vi "WF phase diversity_MATLAB_Correction_loop_AndorSDK_OneCorrApplyToAll_imq.vi"() -> ()   [LabVIEW 2018]
uses:
  <userlib>/WaveKit.lib/Controls/Wavefront Corrector states - ONE.ctl
  <userlib>/WaveKit.lib/Classes/WavefrontCorrector/WavefrontCorrector.lvclass
  <userlib>/WaveKit.lib/Classes/WavefrontCorrectorSet/WavefrontCorrectorSet.lvclass
  <vilib>/Analysis/1siggen.llb/Ramp Pattern by Samples.vi
  <vilib>/Utility/file.llb/Read From Spreadsheet File (DBL).vi
  <vilib>/Analysis/1siggen.llb/Ramp Pattern by Delta.vi
  <vilib>/Analysis/NI_AALBase.lvlib
panel:
  in  "Tab Control":T1(tab)
  in  "Offset command file":path=path "D:/SystemAlignment/system_aberration_20200206.dat"
  in  "Initial haso file":path=path "D:/SystemAlignment/system_aberration_residual_20191015.has"
  out "# of Phase":i32
  in  "Error in":errorcluster
  in  "DM configuration file":path=path "C:/Program Files (x86)/Imagine Optic/Configuration Files/WaveFrontCorrector_mirao52-e_0326.dat"
  out "DM Initial State":T2[](array[typedef])
  out "DM ActuatorsNumber":i32
  out "Error out":errorcluster
  in  "EMCCD trigger port":tag="Dev1/port0/line0"
  in  "Cooler set to Temperature":i32=-60
  in  "Trigger":u32(ring)=1 items=["Internal", "External"]
  out "Return from CheckTimings":u32
  out "Calculated Exposure Value":sgl format="%.2f"
  out "Return from SetTemperature":u32
  out "Cooling":i32
  out "Return from Initialize":u32
  out "Detector X Pixels":i32
  out "Detector Y Pixels":i32
  in  "Initialize EMCCD?":bool=TRUE
  in  "Turn off EMCCD when finished?":bool=TRUE
  in  "Initial Zer coeff":dbl[](array[numeric])=[0.2, 0.2]
  in  "Initial Zer index":dbl[](array[numeric])=[4.0, 5.0]
  out "Initial Zer coeff\nRandomly generated":dbl[](array[numeric])
  out "Initial Zer index (starting from 4)\nrandomly generated":dbl[](array[numeric])
  in  "aberration tolerance":dbl=0.1 format="%#_13g"
  in  "aberration threshold":dbl=0.25 format="%#_13g"
  in  "?":enum16{"input manually ", "randomly generated"}(ring)
  in  "max random order":i64=9
  in  "NOT YET: Data Acquisition Iteration #":i32=1
  in  "Zern index in 2":i32[](array[numeric])=[3, 4, 5, 6, 7, 8]
  in  "Zern coef in 2":sgl[](array[numeric])=[0.0, 0.0, 0.2, 0.0, 0.0, 0.0]
  in  "Zern index in 3":i32[](array[numeric])=[3, 4, 5, 6, 7, 8]
  in  "Zern coef in 3":sgl[](array[numeric])=[0.2, 0.0, 0.0, 0.0, 0.0, 0.0]
  in  "Zern index in 4":i32[](array[numeric])=[3, 4, 5, 6, 7, 8]
  in  "Zern coef in 4":sgl[](array[numeric])=[0.2, 0.0, 0.0, 0.0, 0.0, 0.0]
  in  "Zern index in 5":i32[](array[numeric])=[3, 4, 5, 6, 7, 8]
  in  "Zern coef in 5":sgl[](array[numeric])=[0.0, 0.0, 0.0, 0.0, 0.0, -0.2]
  in  "Andor Picture/notes save to path":path=path "D:/YD/test/test1"
  in  "base name":string="beads_test"
  in  "Pics/phase":dbl=2.0
  in  "camera exposure time (s)":string="0.02"
  in  "# of Phase":i32=5
  in  "COMMAND matrix path":path=path "D:/SystemAlignment/IM_20200224.aomi"
  in  "488 shutter":refnum<k7>(container)
  in  "?":bool
  out "phase diversity file name":string
  out "Corrected Picture name":string
  in  "Z for correction (um) (10 steps=1um)":dbl format="%#_13g"
  in  "ASI stage VISA resource name":refnum<visa-resource-name>="COM5"
  in  "Z scanning range (um)":dbl format="%#_13g"
  in  "Z scanning step (um)":dbl format="%#_13g"
  out "Current Z in step":string="where z"
  in  "Background Value":u32=290
  in  "Run MATLAB or correction?":bool=TRUE
  in  "Keep Reconstructed Defocus component? 2":bool caption="Keep Reconstructed Defocus component?"
  in  "Number for average 2":u32=2
  in  "Zernike Order 2":u32=15
  in  "Iteration Number 2":u32=10
  in  "Gamma Value 2":dbl=1e-06
  in  "Crop Size of image 2":u32=512
  in  "Show Input 2":bool
  in  "Show Recon 2":bool=TRUE
  in  "Use GPU 2":bool=TRUE
  in  "Metrics Type":T3(ring)
  # "If Pics/phase is 2:\npicture order:\n\noffset+aberr *2\nphase diversity *8\n\nground truth *1\noffset+aberr *1\ncorrected *2 but the last one cannot be seen in imagej"
  # "Randomly Generate Initial Zernike, enter here:"
  # "Manually input, enter here:"
  # "Andor Camera Settings"
  # "z-stack is from (Z_for_correction-Z_scanning_range) to (Z_for_correction+Z_scanning_range)"
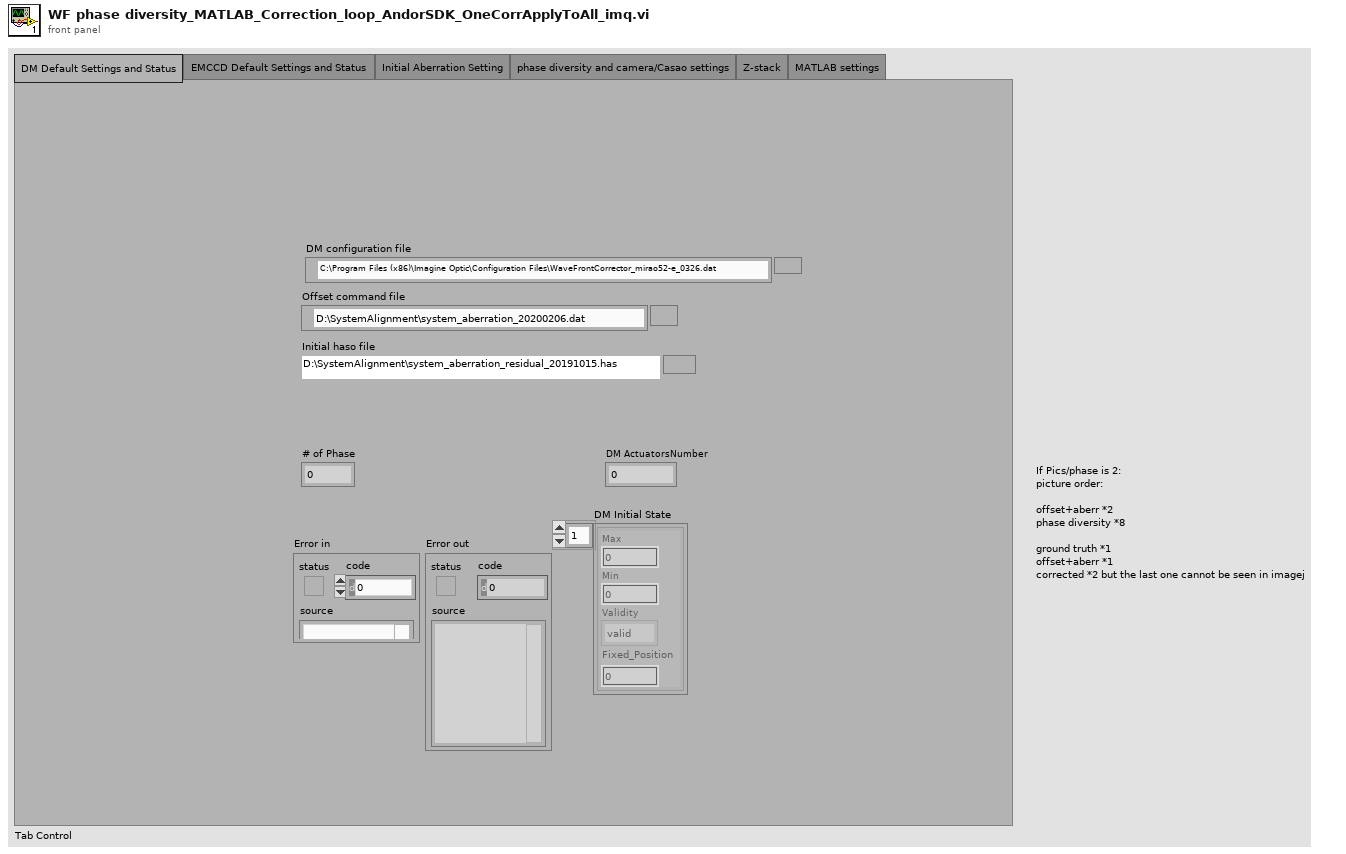
[diagram p1: front panel]
types:
  T1 = enum32{"DM Default Settings and Status", "EMCCD Default Settings and Status ", "Initial Aberration Setting", "phase diversity and camera/Casao settings", "Z-stack", "MATLAB settings"}
  T2 = typedef "Wavefront Corrector states - ONE.ctl" = cluster{"Max":sgl, "Min":sgl, "Validity":enum16{"valid", "fixed", "invalid"}, "Fixed_Position":sgl}
  T3 = enum16{" ", "max intensity", "mean intensity", "RMS contrast", "sharpness - image domain", "sharpness - spectral domain 1: 0~r0", "sharpness - spectral domain 2: 0.1*r0~0.5*r0", "norm DCT  - spectral domain 3: 0~r0"}
  T4 = typedef "Error Code Enum typedef.ctl" = enum32{"N/A (0)", "DRV_ERROR_CODES", "DRV_SUCCESS", "DRV_VXDNOTINSTALLED", "DRV_ERROR_SCAN", "DRV_ERROR_CHECK_SUM", "DRV_ERROR_FILELOAD", "DRV_UNKNOWN_FUNC", "DRV_ERROR_VXD_INIT", "DRV_ERROR_ADDRESS", "DRV_ERROR_PAGELOCK", "DRV_ERROR_PAGEUNLOCK", "DRV_ERROR_BOARDTEST", "DRV_ERROR_ACK", "DRV_ERROR_UP_FIFO", "DRV_ERROR_PATTERN", "N/A (16)", "DRV_ACQUISITION_ERRORS", "DRV_ACQ_BUFFER", "DRV_ACQ_DOWNFIFO_FULL", "DRV_PROC_UNKONWN_INSTRUCTION", "DRV_ILLEGAL_OP_CODE", "DRV_KINETIC_TIME_NOT_MET", "DRV_ACCUM_TIME_NOT_MET", "DRV_NO_NEW_DATA", "N/A (25)", "DRV_SPOOLERROR", "N/A (27)", "N/A (28)", "N/A (29)", "N/A (30)", "N/A (31)", "N/A (32)", "DRV_TEMPERATURE_CODES", "DRV_TEMPERATURE_OFF", "DRV_TEMPERATURE_NOT_STABILIZED", "DRV_TEMPERATURE_STABILIZED", "DRV_TEMPERATURE_NOT_REACHED", "DRV_TEMPERATURE_OUT_RANGE", "DRV_TEMPERATURE_NOT_SUPPORTED", "DRV_TEMPERATURE_DRIFT", "N/A (41)", "N/A (42)", "N/A (43)", "N/A (44)", "N/A (45)", "N/A (46)", "N/A (47)", "N/A (48)", "DRV_GENERAL_ERRORS", "DRV_INVALID_AUX", "DRV_COF_NOTLOADED", "DRV_FPGAPROG", "DRV_FLEXERROR", "DRV_GPIBERROR", "N/A (55)", "N/A (56)", "N/A (57)", "N/A (58)", "N/A (59)", "N/A (60)", "N/A (61)", "N/A (62)", "N/A (63)", "DRV_DATATYPE", "DRV_DRIVER_ERRORS", "DRV_P1INVALID", "DRV_P2INVALID", "DRV_P3INVALID", "DRV_P4INVALID", "DRV_INIERROR", "DRV_COFERROR", "DRV_ACQUIRING", "DRV_IDLE", "DRV_TEMPCYCLE", "DRV_NOT_INITIALIZED", "DRV_P5INVALID", "DRV_P6INVALID", "DRV_INVALID_MODE", "DRV_INVALID_FILTER", "DRV_I2CERRORS", "DRV_I2CDEVNOTFOUND", "DRV_I2CTIMEOUT", "DRV_P7INVALID", "N/A (84)", "N/A (85)", "N/A (86)", "N/A (87)", "N/A (88)", "N/A (89)", "DRV_IOCERROR", "DRV_VRMVERSIONERROR"}
  T5 = typedef "NI_Matrix.lvlib/RealMatrix.ctl" = dbl[][]
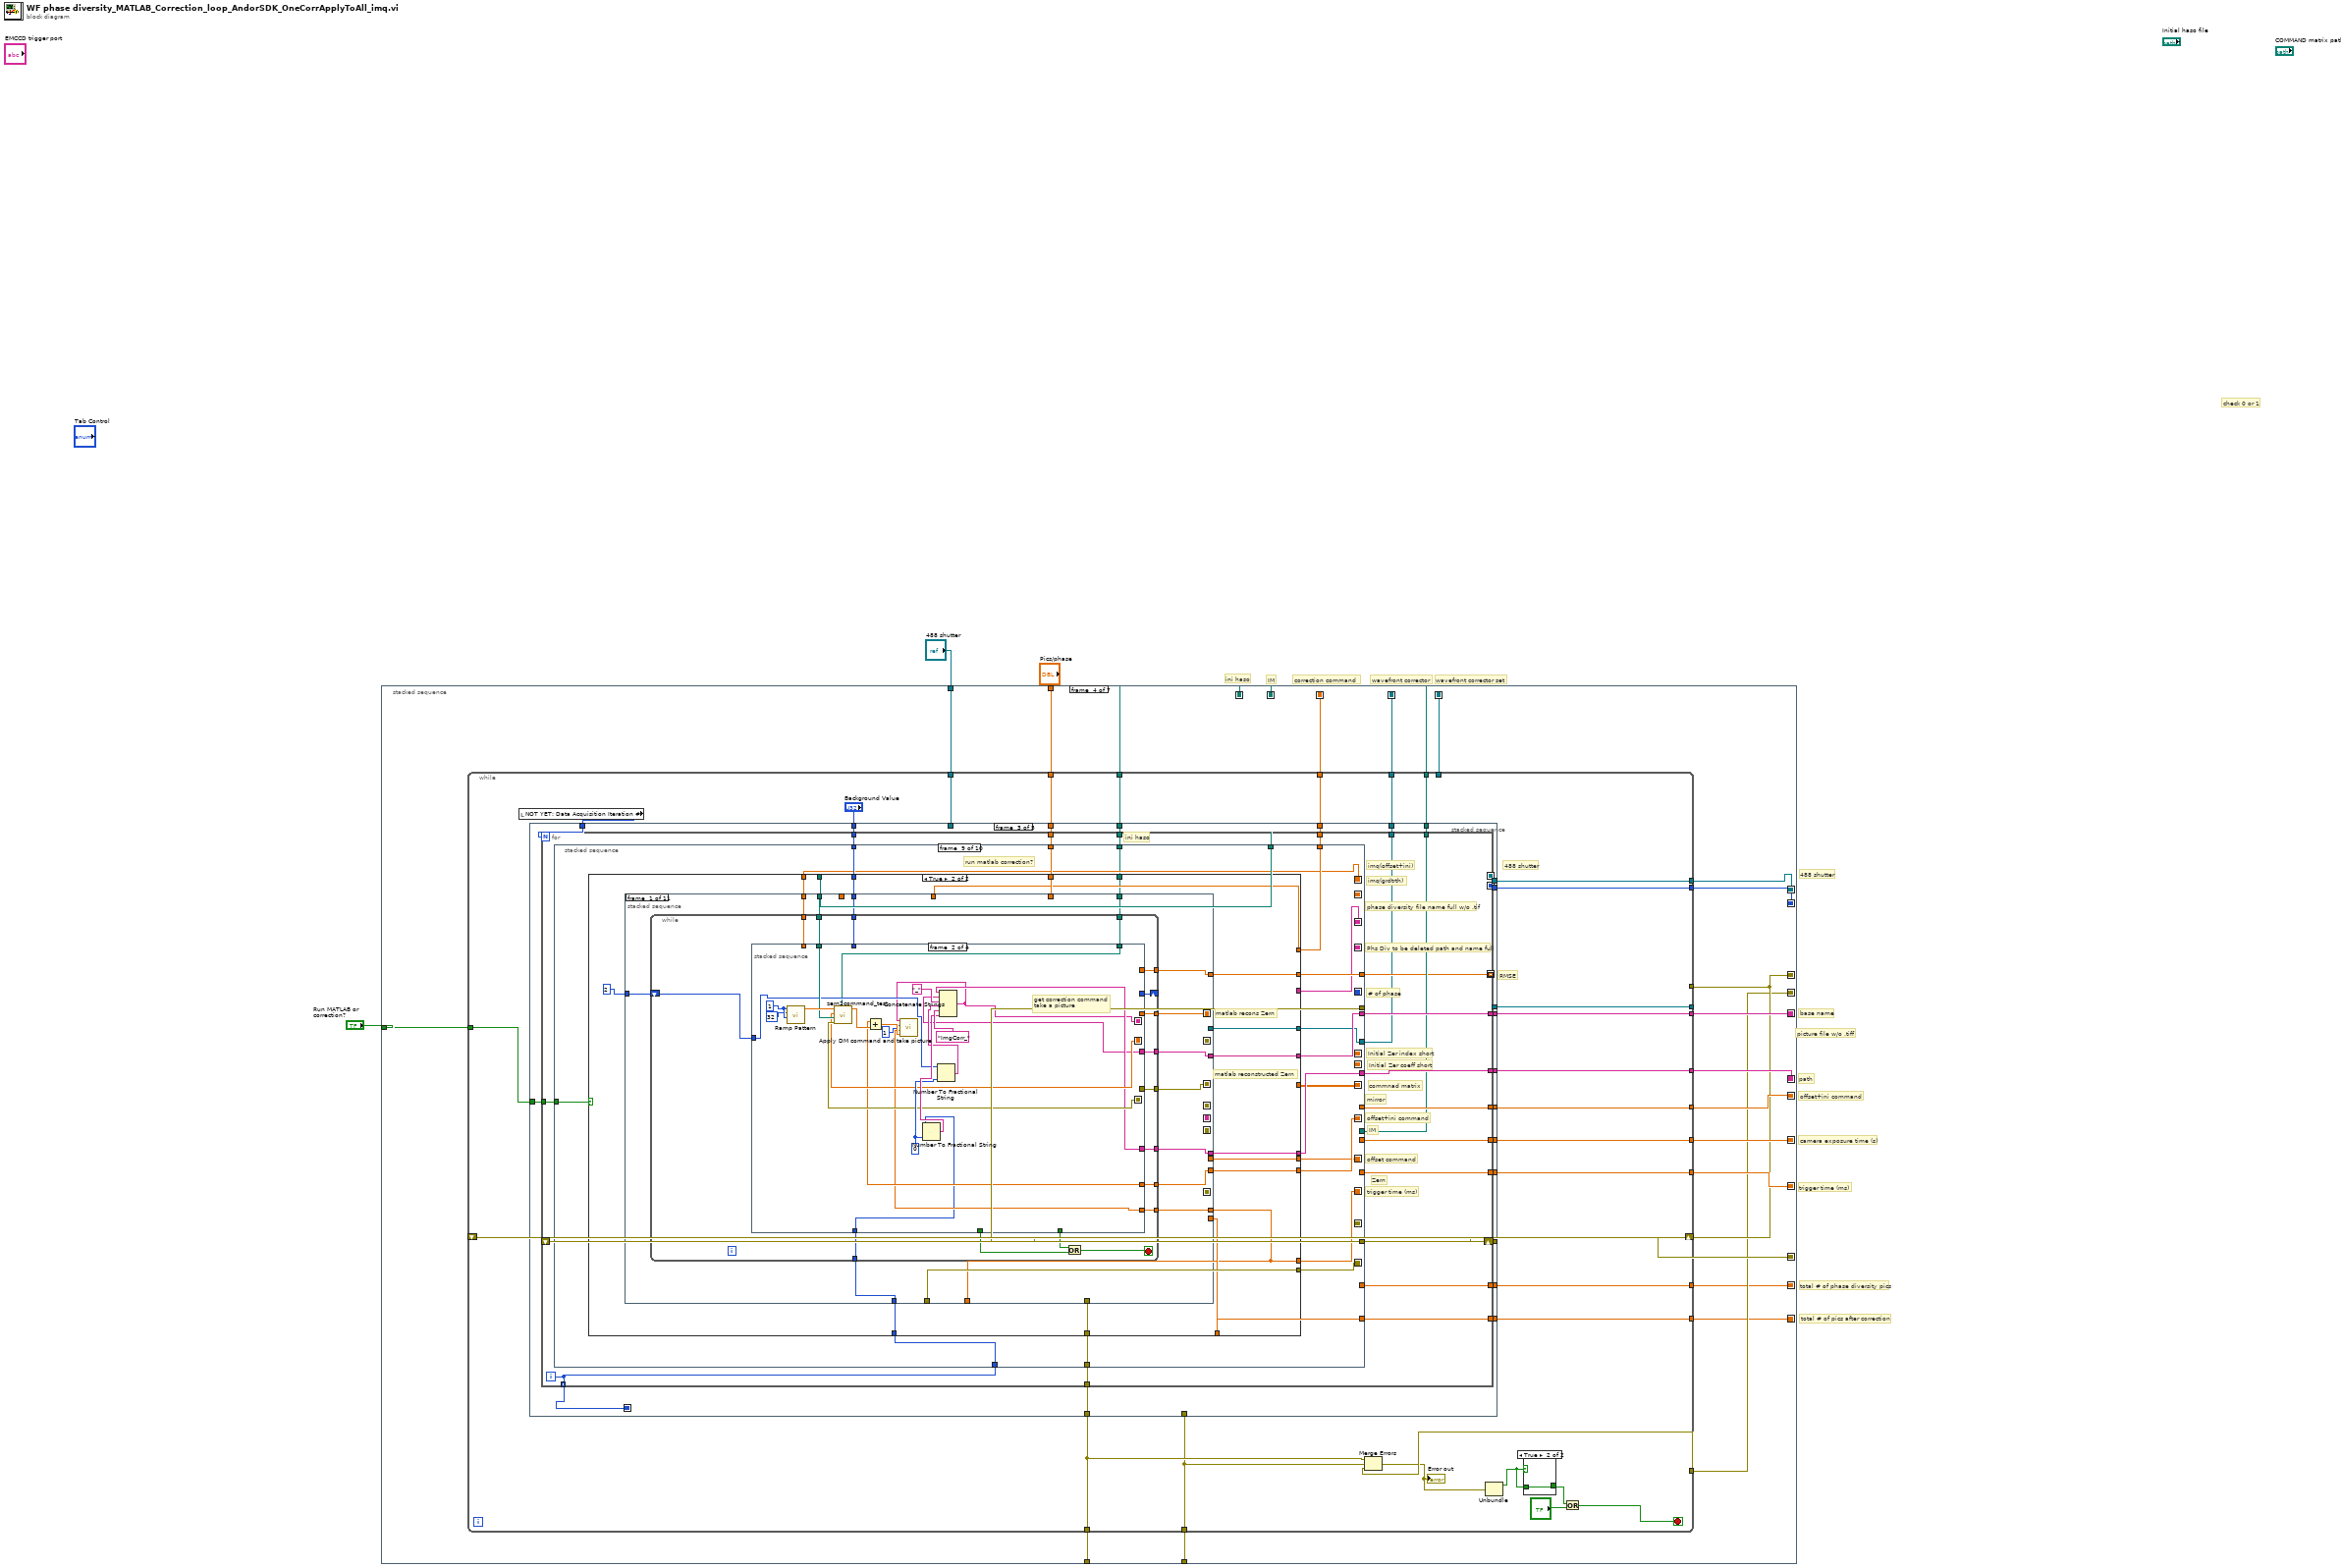
[diagram p0: block diagram]
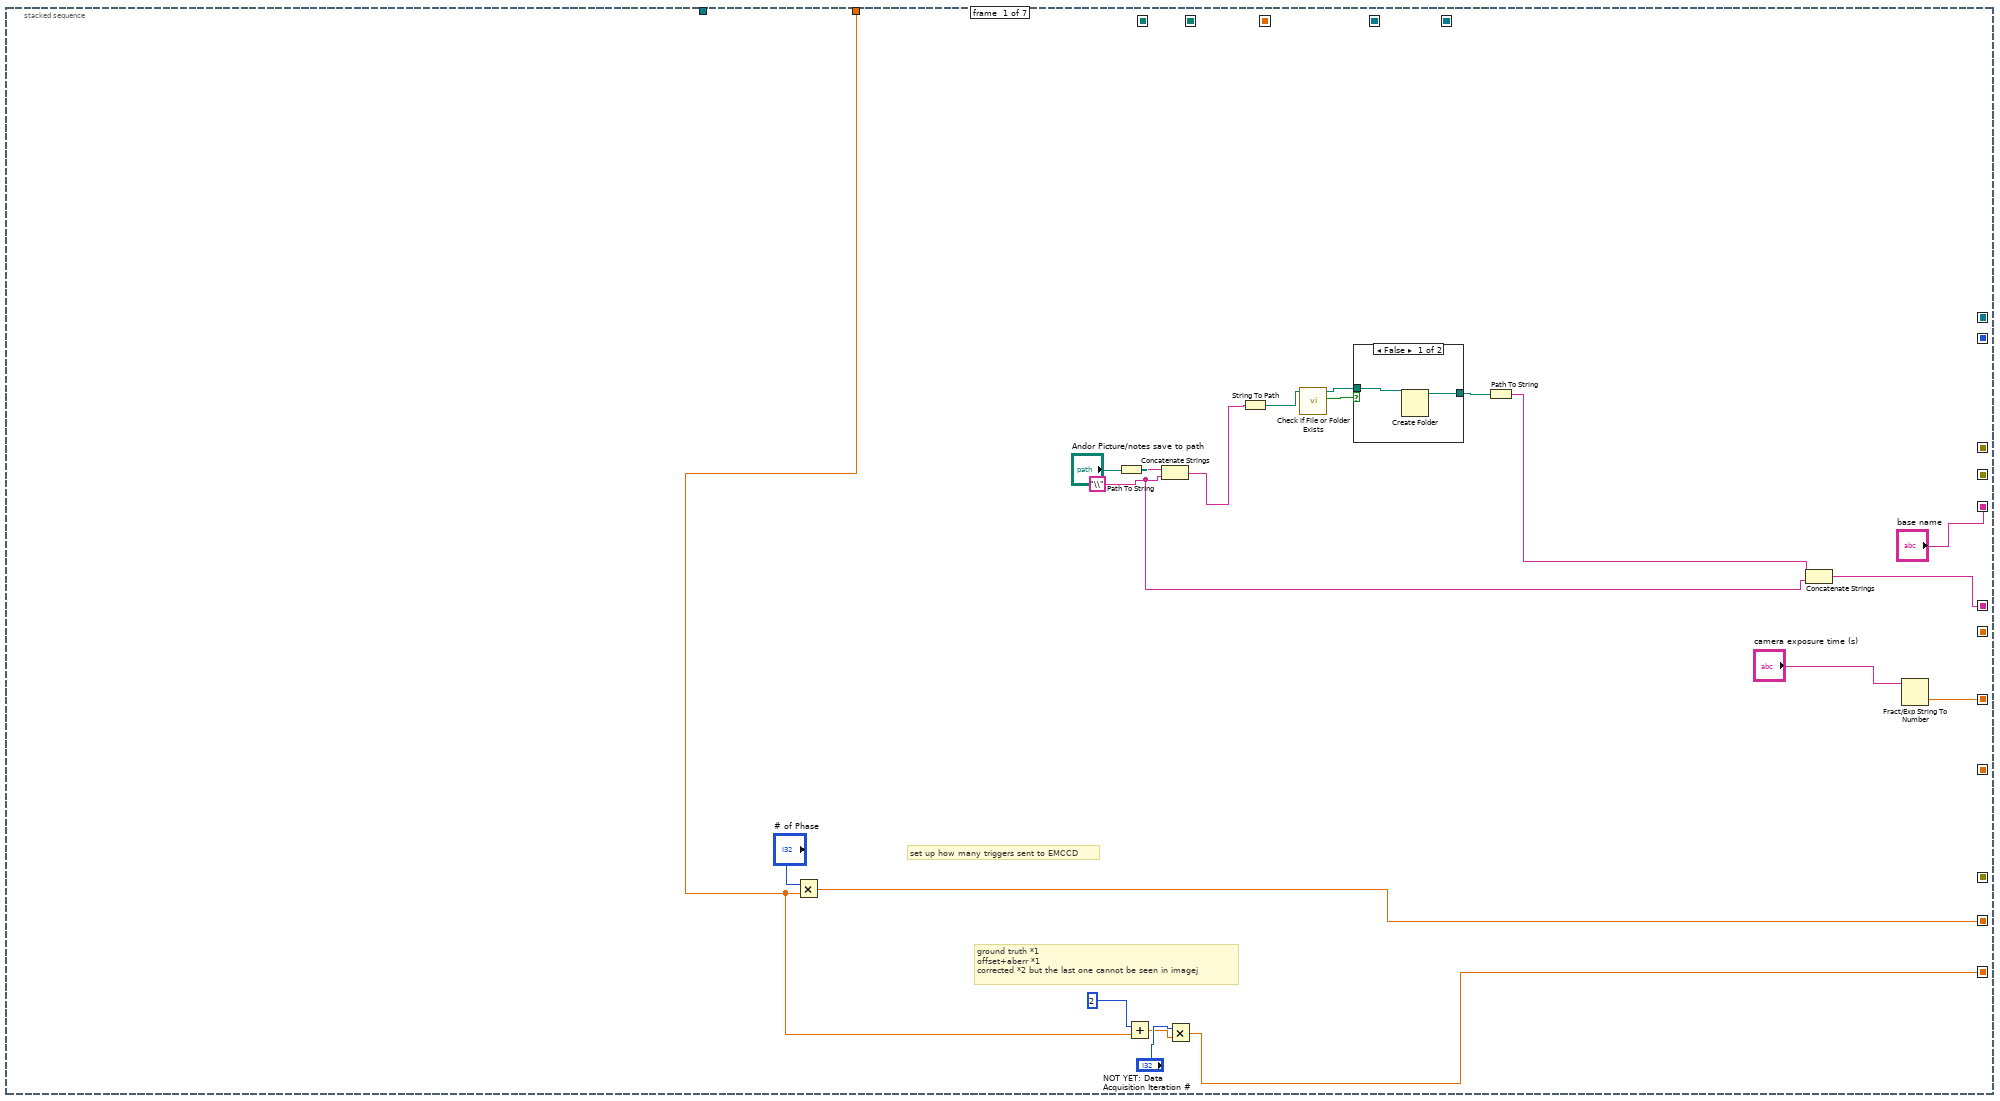
[diagram p2: hidden frame]
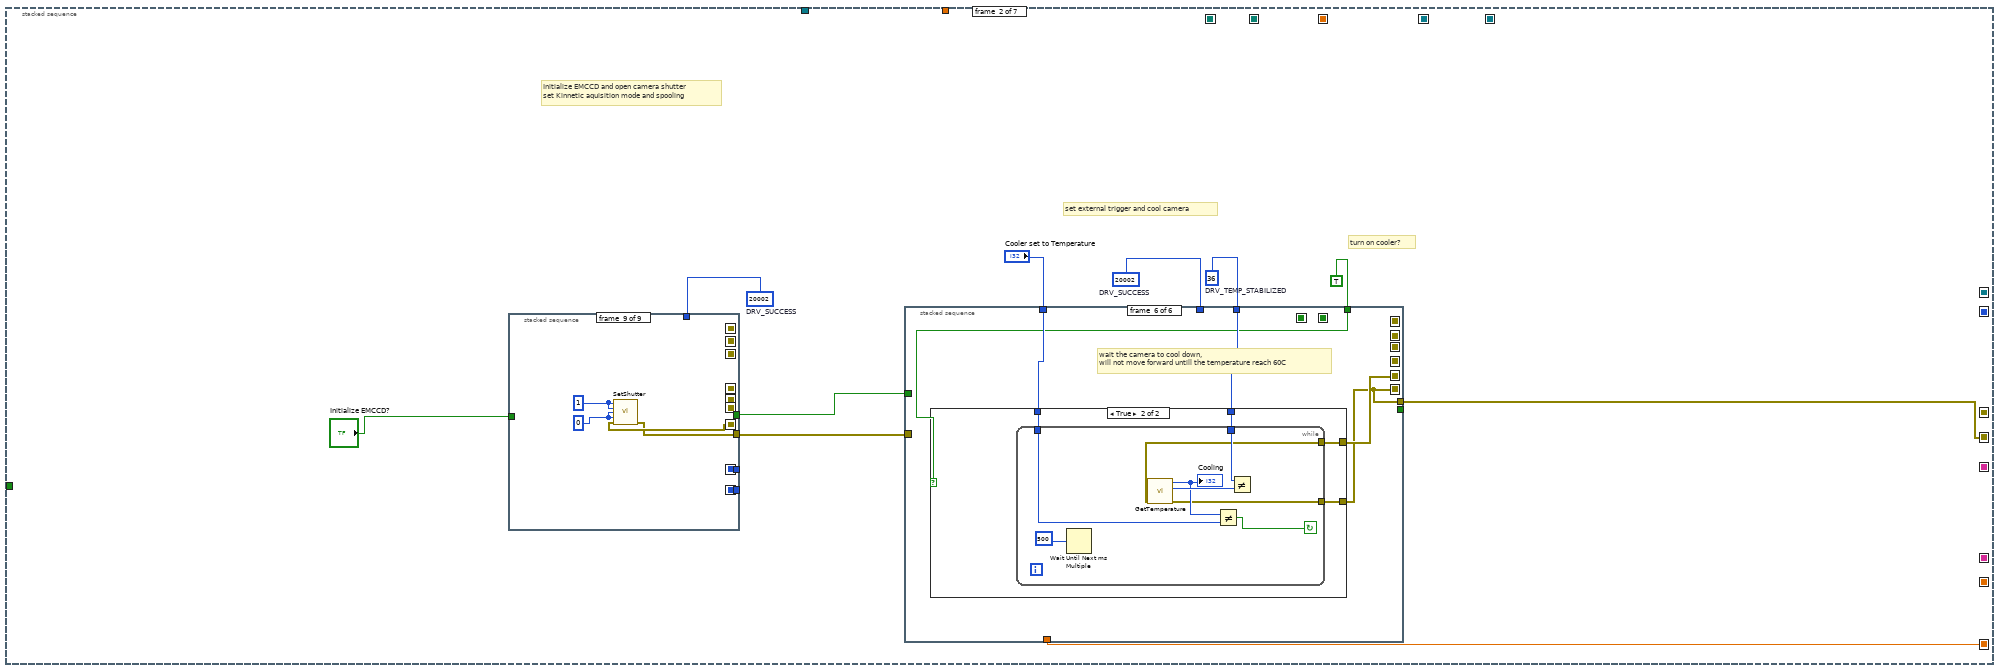
[diagram p4: hidden frame]
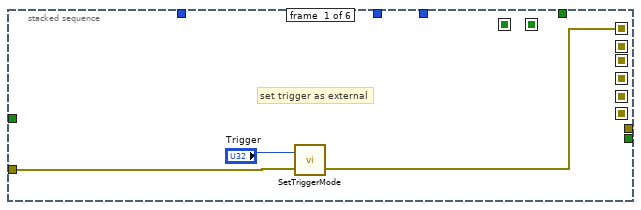
[diagram p5: hidden frame]
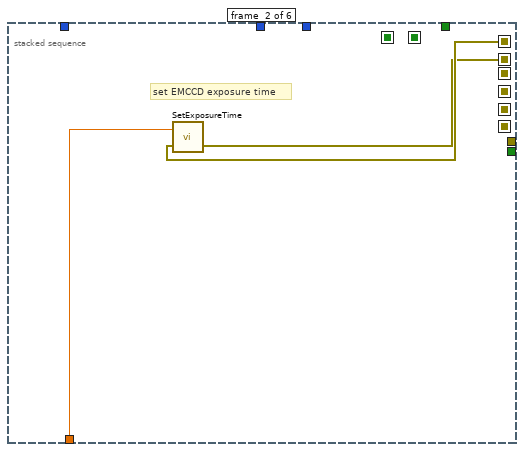
[diagram p6: hidden frame]
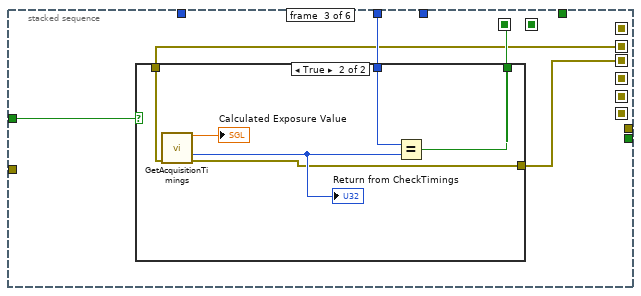
[diagram p7: hidden frame]
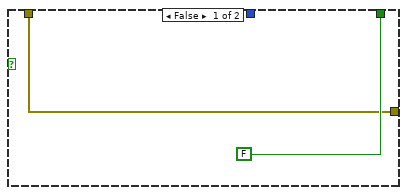
[diagram p8: hidden frame]
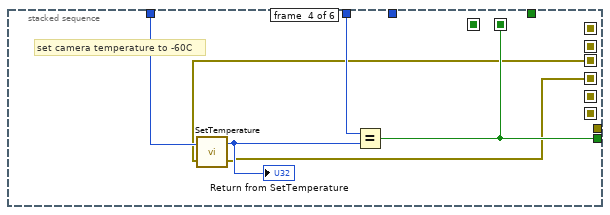
[diagram p9: hidden frame]
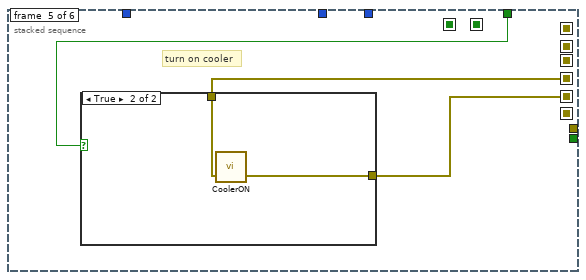
[diagram p10: hidden frame]
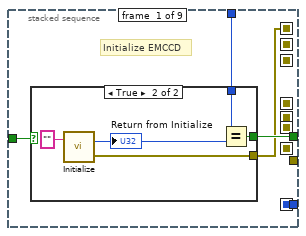
[diagram p13: hidden frame]
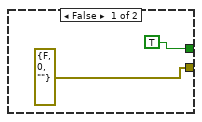
[diagram p14: hidden frame]
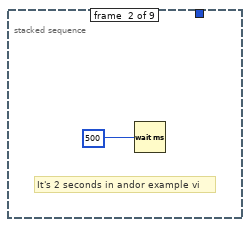
[diagram p15: hidden frame]
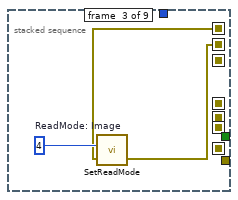
[diagram p16: hidden frame]
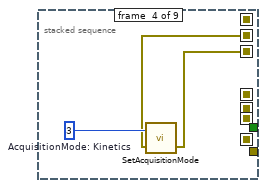
[diagram p17: hidden frame]
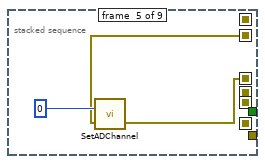
[diagram p18: hidden frame]
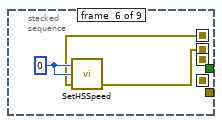
[diagram p19: hidden frame]
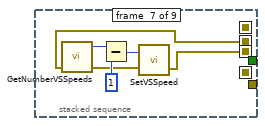
[diagram p20: hidden frame]
diagram:
  # "correction command"
  # "total # of phase diversity pics"
  # "picture file w/o .tiff"
  # "total # of pics after correction"
  # "wavefront corrector set"
  # "wavefront corrector"
  # "488 shutter"
  # "trigger time (ms)"
  # "offset+ini command"
  # "camera exposure time (s)"
  # "IM"
  # "ini haso"
  # "path"
  # "base name"
  # "check 0 or 1"
  n1 = stacked-sequence {
    seq-local: [w4 _ _ _ _ _ _] -> [_ _ _ w165 w746 _ _]
    seq-local: ["base name" _ _ _ _ _ _] -> [_ _ _ w164 w745 _ _]
    seq-local: [_ _ w144 _ _ _ _] -> [_ _ _ w163 _ _ _]
    seq-local: [_ _ w143 _ _ _ _] -> [_ _ _ w158 _ _ _]
    seq-local: [w18 _ _ _ _ _ _] -> [_ w29 _ w162 _ _ _]
    seq-local: [_ _ w128 _ _ _ _] -> [_ _ _ w150 _ _ _]
    seq-local: [_ _ _ w161 _ _ _] -> [_ _ _ _ _ _ _]
    seq-local: [_ _ _ w160 _ _ _] -> [_ _ _ _ w742 _ _]
    seq-local: [_ _ _ w159 _ _ _] -> [_ _ _ _ _ _ w828]
    seq-local: [_ _ _ w153 _ _ _] -> [_ _ _ _ w754 _ _]
    seq-local: [_ _ _ w156 _ _ _] -> [_ _ _ _ w753 _ _]
    seq-local: [_ _ w127 _ _ _ _] -> [_ _ _ w151 w751 _ w830]
    seq-local: [_ _ w126 _ _ _ _] -> [_ _ _ w149 _ _ w829]
    seq-local: [w15 _ _ _ _ _ _] -> [_ _ _ w146 _ _ _]
    seq-local: [_ w30 _ _ _ _ _] -> [_ _ _ w148 _ _ _]
    seq-local: [w14 _ _ _ _ _ _] -> [_ _ _ w147 _ _ _]
    seq-local: [_ _ _ w145 _ _ _] -> [_ _ _ _ w752 _ _]
    tunnel: "Pics/phase" -> [w12 _ _ w166 _ _ _]
    tunnel: "Run MATLAB or correction?" -> [_ _ _ w157 _ _ _]
    tunnel: [_ _ _ w155 _ _ _] -> _
    tunnel: [_ _ _ w154 _ _ _] -> _
    tunnel: "488 shutter" -> [_ _ _ w152 _ _ w831]
    frame #0 {
      w5 = "\\"
      # "set up how many triggers sent to EMCCD"
      # "ground truth *1\noffset+aberr *1\ncorrected *2 but the last one cannot be seen in imagej"
      n2 = Multiply(x="# of Phase", y=w12) -> (x*y=w14:dbl)
      n3 = Path To String(path="Andor Picture/notes save to path") -> (string=w20:string)
      n4 = Add(x=2, y=w12) -> (x+y=w16:dbl)
      n5 = Concatenate Strings(w20, w5) -> (w7:string)
      n6 = Multiply(x="NOT YET: Data Acquisition Iteration #", y=w16) -> (x*y=w15:dbl)
      n7 = String To Path(string=w7) -> (path=w11:path)
      n8 = call <vilib>:"Check if File or Folder Exists.vi"("path"=w11) -> ("file or folder exists?"=w9:bool, "dup path"=w10:path)  [unwired: 8 in, 1 out]
      n9 = case shown="False" w9 {
        tunnel: w10 -> [w25 w26]
        tunnel: [w24 w26] -> w8
        frame False {
          n10 = Create Folder(path (use dialog)=w25) -> (created path=w24:path)  [unwired: 2 in, 2 out]
        }
        frame True {
        }
      }
      n11 = Path To String(path=w8) -> (string=w6:string)
      n12 = Concatenate Strings(w6, w5) -> (w4:string)
      n13 = Fract/Exp String To Number(string="camera exposure time (s)") -> (number=w18:dbl)  [unwired: 3 in, 1 out]
    }
    frame #1 {
      w32 = 36  # DRV_TEMP_STABILIZED
      w34 = 20002  # DRV_SUCCESS
      w36 = 20002  # DRV_SUCCESS
      # "turn on cooler?"
      # "set external trigger and cool camera"
      # "Initialize EMCCD and open camera shutter\nset Kinnetic aquisition mode and spooling"
      n14 = stacked-sequence {
        seq-local: [_ _ _ _ _ _ _ w120 _] -> [_ _ _ _ _ _ _ _ _]
        seq-local: [_ _ _ _ _ _ _ w119 _] -> [_ _ _ _ _ _ _ _ _]
        seq-local: [w87 _ _ _ _ _ _ _ _] -> [_ _ w99 _ _ _ _ _ _]
        seq-local: [_ _ w98 _ _ _ _ _ _] -> [_ _ _ w102 _ _ _ _ _]
        seq-local: [_ _ _ w101 _ _ _ _ _] -> [_ _ _ _ w104 _ _ _ _]
        seq-local: [_ _ _ _ w105 _ _ _ _] -> [_ _ _ _ _ w108 _ _ _]
        seq-local: [_ _ _ _ _ w107 _ _ _] -> [_ _ _ _ _ _ w112 _ _]
        seq-local: [_ _ _ _ _ _ w110 _ _] -> [_ _ _ _ _ _ _ w118 _]
        seq-local: [_ _ _ _ _ _ _ w116 _] -> [_ _ _ _ _ _ _ _ w123]
        tunnel: w36 -> [w89 _ _ _ _ _ _ _ _]
        tunnel: [w88 _ _ _ _ _ _ _ _] -> w35
        tunnel: [_ _ _ _ _ _ _ w120 _] -> _
        tunnel: [_ _ _ _ _ _ _ w119 _] -> _
        tunnel: [_ _ _ _ _ _ _ _ w122] -> w31
        tunnel: "Initialize EMCCD?" -> [w86 _ _ _ _ _ _ _ _]
        frame #0 {
          # "Initialize EMCCD"
          n15 = case shown="True" w86 {
            tunnel: w89 -> [_ w94]
            tunnel: [TRUE w93] -> w88
            tunnel: [errorcluster {"status"=FALSE, "code"=0, "source"=""} ("Error in 2") w92] -> w87
            frame False {
            }
            frame True {
              n16 = call <userlib>:"Initialize.vi"("directory (\"\")"="" ("directory (\"\")")) -> ("error out"=w92:errorcluster, "DLL error code"=w96:u32)  [unwired: 1 in]
              "Return from Initialize" <- w96
              n17 = Equal?(x=w94, y=w96) -> (x = y?=w93:bool)
            }
          }
        }
        frame #1 {
          # "It's 2 seconds in andor example vi"
          n18 = Wait (ms)(milliseconds to wait=u32 500) -> ()  [unwired: 1 out]
        }
        frame #2 {
          w100 = u16 4  # ReadMode: Image
          n19 = call <userlib>:"SetReadMode.vi"("error in (no error)"=w99, "mode"=w100) -> ("error out"=w98:errorcluster)  [unwired: 1 out]
        }
        frame #3 {
          w103 = u16 3  # AcquisitionMode: Kinetics
          n20 = call <userlib>:"SetAcquisitionMode.vi"("error in (no error)"=w102, "mode"=w103) -> ("error out"=w101:errorcluster)  [unwired: 1 out]
        }
        frame #4 {
          n21 = call <userlib>:"SetADChannel.vi"("error in (no error)"=w104, "channel"=0) -> ("error out"=w105:errorcluster)  [unwired: 1 out]
        }
        frame #5 {
          w109 = 0
          n22 = call <userlib>:"SetHSSpeed.vi"("error in (no error)"=w108, "index"=w109, "type"=w109) -> ("error out"=w107:errorcluster)  [unwired: 1 in, 1 out]
        }
        frame #6 {
          n23 = call <userlib>:"GetNumberVSSpeeds.vi"("error in (no error)"=w112) -> ("error out"=w111:errorcluster, "number"=w115:i32)  [unwired: 2 in, 1 out]
          n24 = Subtract(x=w115, y=1) -> (x-y=w113:i32)
          n25 = call <userlib>:"SetVSSpeed.vi"("error in (no error)"=w111, "index"=w113) -> ("error out"=w110:errorcluster)  [unwired: 1 out]
        }
        frame #7 {
          w121 = 1
          n26 = call <userlib>:"GetDetector.vi"("error in (no error)"=w118) -> ("error out"=w117:errorcluster, "ypixels"=w120:i32, "xpixels"=w119:i32)  [unwired: 3 in, 1 out]
          "Detector Y Pixels" <- w120
          "Detector X Pixels" <- w119
          n27 = call <userlib>:"SetImage.vi"("hbin"=w121, "vbin"=w121, "hstart"=w121, "hend"=w119, "vstart"=w121, "vend"=w120, "error in (no error)"=w117) -> ("error out"=w116:errorcluster)  [unwired: 19 in, 1 out]
        }
        frame #8 {
          w124 = 0
          w125 = 1
          n28 = call <userlib>:"SetShutter.vi"("type"=w125, "mode"=w125, "closingtime"=w124, "openingtime"=w124, "error in (no error)"=w123) -> ("error out"=w122:errorcluster)  [unwired: 9 in, 1 out]
        }
      }
      n29 = stacked-sequence {
        seq-local: [_ _ w45 _ _ _] -> [_ _ _ _ _ _]
        seq-local: [_ _ _ w58 _ _] -> [_ _ _ _ _ _]
        seq-local: [w37 _ _ _ _ _] -> [_ w42 _ _ _ _]
        seq-local: [_ w41 _ _ _ _] -> [_ _ w44 _ _ _]
        seq-local: [_ _ w43 _ _ _] -> [_ _ _ w57 _ _]
        seq-local: [_ _ _ w56 _ _] -> [_ _ _ _ w64 _]
        seq-local: [_ _ _ _ w63 _] -> [_ _ _ _ _ w70]
        seq-local: [_ _ _ _ _ w68] -> [_ _ _ _ _ _]
        tunnel: w34 -> [_ _ w47 w61 _ _]
        tunnel: "Cooler set to Temperature" -> [_ _ _ w59 _ w71]
        tunnel: w32 -> [_ _ _ _ _ w72]
        tunnel: [_ _ _ w58 _ _] -> _
        tunnel: w35 -> [_ _ w46 _ _ _]
        tunnel: w31 -> [w38 _ _ _ _ _]
        tunnel: [_ _ _ _ _ w68] -> w30
        tunnel: w29 -> [_ w40 _ _ _ _]
        tunnel: TRUE -> [_ _ _ _ w62 w69]
        frame #0 {
          # "set trigger as external"
          n30 = call <userlib>:"SetTriggerMode.vi"("error in (no error)"=w38, "mode"="Trigger") -> ("error out"=w37:errorcluster)  [unwired: 1 out]
        }
        frame #1 {
          # "set EMCCD exposure time"
          n31 = call <userlib>:"SetExposureTime.vi"("error in (no error)"=w42, "time"=w40) -> ("error out"=w41:errorcluster)  [unwired: 1 out]
        }
        frame #2 {
          n32 = case shown="True" w46 {
            tunnel: w47 -> [_ w53]
            tunnel: [FALSE w55] -> w45
            tunnel: w44 -> [w48 w51]
            tunnel: [w48 w50] -> w43
            frame False {
            }
            frame True {
              n33 = call <userlib>:"GetAcquisitionTimings.vi"("error in (no error)"=w51) -> ("exposure"=→"Calculated Exposure Value":sgl, "DLL error code"=w52:u32, "error out"=w50:errorcluster)  [unwired: 10 in, 2 out]
              "Return from CheckTimings" <- w52
              n34 = Equal?(x=w53, y=w52) -> (x = y?=w55:bool)
            }
          }
        }
        frame #3 {
          # "set camera temperature to -60C"
          n35 = call <userlib>:"SetTemperature.vi"("error in (no error)"=w57, "temperature"=w59) -> ("error out"=w56:errorcluster, "DLL error code"=w60:u32)
          "Return from SetTemperature" <- w60
          n36 = Equal?(x=w61, y=w60) -> (x = y?=w58:bool)
        }
        frame #4 {
          # "turn on cooler"
          n37 = case shown="True" w62 {
            tunnel: w64 -> [w65 w67]
            tunnel: [w65 w66] -> w63
            frame False {
            }
            frame True {
              n38 = call <userlib>:"CoolerON.vi"("error in (no error)"=w67) -> ("error out"=w66:errorcluster)  [unwired: 1 in, 1 out]
            }
          }
        }
        frame #5 {
          # "wait the camera to cool down,\nwill not move forward untill the temperature reach 60C"
          n39 = case shown="True" w69 {
            tunnel: w72 -> [_ w77]
            tunnel: w71 -> [_ w76]
            tunnel: w70 -> [w73 w75]
            tunnel: [w73 w74] -> w68
            frame False {
            }
            frame True {
              n40 = while {
                tunnel: w77 -> [w84]
                tunnel: w76 -> [w81]
                tunnel: w75 -> [w79]
                tunnel: [w78] -> w74
                stop <- w80 continue-if-true
                n41 = Wait Until Next ms Multiple(millisecond multiple=u32 500) -> ()  [unwired: 1 out]
                n42 = call <userlib>:"GetTemperature.vi"("error in (no error)"=w79) -> ("error out"=w78:errorcluster, "status"=w83:T4, "temperature"=w82:i32)  [unwired: 3 in, 1 out]
                "Cooling" <- w82
                n43 = Not Equal?(x=w82, y=w81) -> (x != y?=w80:bool)
                n44 = Not Equal?(x=w84, y=w83) -> ()  [unwired: 1 out]
              }
            }
          }
        }
      }
    }
    frame #2 {
      # "Initialize CASAO"
      n45 = call <userlib>:"LVClass_WavefrontCorrectorSet ctor.vi"("WavefrontCorrectorSet in"=refnum<class "WavefrontCorrectorSet.lvclass"> refnum, "PathToWavefrontCorrectorSetupFile"="DM configuration file", "error in (no error)"="Error in") -> ("WavefrontCorrectorSet out"=w133:refnum<class "WavefrontCorrectorSet.lvclass">, "error out"=w142:errorcluster)  [unwired: 11 in]
      n46 = call <userlib>:"LVClass_WavefrontCorrector ctor.vi"("WavefrontCorrector in"=refnum<class "WavefrontCorrector.lvclass"> refnum, "PathToWavefrontCorrectorSetupFile"="DM configuration file", "error in (no error)"=w142) -> ("WavefrontCorrector out"=w137:refnum<class "WavefrontCorrector.lvclass">, "error out"=w136:errorcluster)  [unwired: 11 in]
      n47 = call <userlib>:"LVClass_WavefrontCorrector Init.vi"("WavefrontCorrector in"=w137, "set_init_state_from_config_file"=TRUE, "error in (no error)"=w136) -> ("WavefrontCorrector out"=w131:refnum<class "WavefrontCorrector.lvclass">, "error out"=w135:errorcluster)  [unwired: 11 in]
      n48 = call <userlib>:"LVClass_WavefrontCorrectorSet get nb of actuators.vi"("WavefrontCorrectorSet in"=w133, "error in (no error)"=w135) -> ("WavefrontCorrectorSet out"=w126:refnum<class "WavefrontCorrectorSet.lvclass">, "ActuatorsNumber"=→"DM ActuatorsNumber":i32, "error out"=w132:errorcluster)  [unwired: 11 in]
      n49 = call <userlib>:"LVClass_WavefrontCorrector Get Current Preferences.vi"("WavefrontCorrector in"=w131, "error in (no error)"=w132) -> ("WavefrontCorrector out"=w127:refnum<class "WavefrontCorrector.lvclass">, "Mirror preferences.Wavefront Corrector State"=→"DM Initial State":T2[], "error out"=w128:errorcluster)  [unwired: 10 in, 1 out]
      n50 = local read "COMMAND matrix path"() -> (w143:path)
      n51 = local read "Initial haso file"() -> (w144:path)
    }
    frame #3 {
      n52 = while {
        tunnel: w166 -> [w195]
        tunnel: w165 -> [w194]
        tunnel: w164 -> [w193]
        tunnel: w163 -> [w192]
        tunnel: w162 -> [w191]
        tunnel: [w189] -> w161
        tunnel: [w188] -> w160
        tunnel: w158 -> [w186]
        tunnel: w157 -> [w185]
        tunnel: [w184] -> w156
        tunnel: [w183] -> _
        tunnel: [w181] -> w155
        tunnel: [w182] -> w154
        shift-right: [w187] -> w159
        shift-left: w150 -> [w190]
        tunnel: [w180] -> w153
        tunnel: w152 -> [w179]
        tunnel: w151 -> [w178]
        tunnel: w150 -> [_]
        tunnel: w149 -> [_]
        tunnel: w148 -> [w176]
        tunnel: w147 -> [w170]
        tunnel: w146 -> [w169]
        tunnel: [w168] -> w145
        stop <- w172 stop-if-true
        # "488 shutter"
        # "RMSE"
        n53 = local read "NOT YET: Data Acquisition Iteration #"() -> (w177:i32)
        n54 = stacked-sequence {
          seq-local: [_ _ w220 _ _] -> [_ _ _ _ w737]
          seq-local: [_ _ w219 _ _] -> [_ _ _ _ _]
          seq-local: [_ w207 _ _ _] -> [_ _ _ w733 _]
          seq-local: [_ w208 _ _ _] -> [_ _ _ w732 _]
          tunnel: w195 -> [_ _ w232 _ _]
          tunnel: w194 -> [_ _ w231 _ w736]
          tunnel: w193 -> [_ _ w230 _ w735]
          tunnel: w192 -> [_ _ w229 _ _]
          tunnel: w191 -> [_ _ w228 _ _]
          tunnel: w190 -> [_ _ w227 _ _]
          tunnel: [_ _ w226 _ _] -> w189
          tunnel: [_ _ w225 _ _] -> w188
          tunnel: [_ _ w224 _ _] -> w187
          tunnel: w186 -> [_ _ w223 _ _]
          tunnel: w185 -> [_ _ w222 _ _]
          tunnel: w177 -> [_ _ w221 _ _]
          tunnel: [_ _ _ w731 _] -> w183
          tunnel: [_ _ _ w730 _] -> w184
          tunnel: [_ _ _ _ w734] -> w181
          tunnel: [_ _ w218 _ _] -> w182
          tunnel: [_ w207 _ _ _] -> w180
          tunnel: w179 -> [_ w206 _ _ _]
          tunnel: w178 -> [_ _ w217 _ _]
          tunnel: w170 -> [_ _ w216 _ _]
          tunnel: w169 -> [_ _ w215 _ _]
          tunnel: [_ _ w214 _ _] -> w168
          tunnel: "Background Value" -> [_ _ w213 _ _]
          frame #0 {
            # "10 step=1um"
            # "MOVE TO Z FOR CORRECTION"
            n55 = Multiply(x="Z for correction (um) (10 steps=1um)", y=10.0) -> (x*y=w199:dbl)
            n56 = local read "ASI stage VISA resource name"() -> (w202:refnum<visa-resource-name>)
            n57 = Number To Decimal String(number=w199) -> (decimal integer string=w204:string)  [unwired: 1 in]
            n58 = Concatenate Strings("move z=", w204) -> (w203:string)
            n59 = call "WriteCmd.vi"("Command"=w203, "VISA resource name"=w202) -> ()  [unwired: 1 in, 1 out]
          }
          frame #1 {
            # "open the shutter of 488nm laser"
            n60 = property class="MG17Motor"(reference=w206, "HWSerialNum"=85819115.0) -> (reference out=w212:refnum<k7>)  [unwired: 1 in, 1 out]
            n61 = invoke class="MG17Motor" method="StartCtrl"(reference=w212) -> (reference out=w210:refnum<k7>)  [unwired: 2 in, 2 out]
            n62 = invoke class="MG17Motor" method="SC_Enable"(reference=w210, "lChanID"=0) -> (reference out=w207:refnum<k7>, "lChanID"=w208:i32)  [unwired: 2 in, 2 out]
          }
          frame #2 {
            n63 = for {
              N: w221 -> [_]
              tunnel: w232 -> [w251]
              tunnel: w231 -> [w250]
              tunnel: w230 -> [w249]
              tunnel: w229 -> [w248]
              tunnel: w228 -> [w247]
              tunnel: [w245] -> w226
              tunnel: [w244] -> w225
              tunnel: w223 -> [w242]
              tunnel: w222 -> [w241]
              shift-right: [w243] -> w224
              shift-left: w227 -> [w246]
              tunnel: [w240] -> w220 mode=indexing
              tunnel: [w239] -> w219 mode=indexing
              tunnel: [w238] -> w218
              tunnel: w217 -> [w237]
              tunnel: w216 -> [w236]
              tunnel: w215 -> [w235]
              tunnel: [w234] -> w214
              tunnel: w213 -> [w233]
              i -> [w239]
              # "imq(grdtrth)"
              # "imq(offset+ini)"
              # "Phs Div to be deleted path and name full"
              # "phase diversity file name full w/o .tif"
              # "# of phase"
              # "trigger time (ms)"
              # "offset+ini command"
              # "Initial Zer coeff short"
              # "Initial Zer index short"
              # "mirror"
              # "Zern"
              # "commnad matrix"
              # "ini haso"
              # "IM"
              # "offset command"
              n64 = stacked-sequence {
                seq-local: [_ w263 _ _ _ _ _ _ _ _] -> [_ _ w283 _ w411 _ _ w464 w512 _]
                seq-local: [_ _ w281 _ _ _ _ _ _ _] -> [_ _ _ _ w410 _ _ _ w514 _]
                seq-local: [_ _ w279 _ _ _ _ _ _ _] -> [_ _ _ _ w409 _ _ _ _ _]
                seq-local: [_ _ w272 _ _ _ _ _ _ _] -> [_ _ _ _ w406 _ _ _ _ _]
                seq-local: [w254 _ _ _ _ _ _ _ _ _] -> [_ _ w269 _ _ _ _ _ _ _]
                seq-local: [w253 _ _ _ _ _ _ _ _ _] -> [_ _ w268 _ _ _ _ _ _ _]
                seq-local: [_ _ w267 _ _ _ _ _ _ _] -> [_ _ _ _ _ _ _ w462 w520 _]
                seq-local: [_ _ _ _ w405 _ _ _ _ _] -> [_ _ _ _ _ w446 _ w463 w518 _]
                seq-local: [_ _ _ _ w404 _ _ _ _ _] -> [_ _ _ _ _ _ _ _ w517 _]
                seq-local: [_ _ _ _ _ _ w449 _ _ _] -> [_ _ _ _ _ _ _ _ w508 _]
                seq-local: [_ _ _ w398 _ _ _ _ _ _] -> [_ _ _ _ _ _ _ _ _ w719]
                seq-local: [_ _ _ _ _ _ _ w461 _ _] -> [_ _ _ _ _ _ _ _ w505 _]
                seq-local: [_ _ _ _ _ _ _ w460 _ _] -> [_ _ _ _ _ _ _ _ _ _]
                tunnel: w251 -> [_ _ w276 _ w414 _ _ _ w519 _]
                tunnel: w250 -> [_ _ w277 w401 w413 _ w457 w468 w522 _]
                tunnel: w249 -> [_ _ w278 w400 w412 _ w459 w467 w523 _]
                tunnel: w248 -> [_ _ w275 _ _ _ _ _ w504 _]
                tunnel: w242 -> [_ _ w274 _ w408 _ _ _ _ _]
                tunnel: w247 -> [_ _ _ _ w407 _ _ _ _ _]
                tunnel: w246 -> [_ _ w273 _ _ _ _ _ _ _]
                tunnel: [_ _ _ _ w404 _ _ _ _ _] -> w243
                tunnel: [_ _ w267 _ _ _ _ _ _ _] -> w245
                tunnel: [_ _ _ _ w405 _ _ _ _ _] -> w244
                tunnel: w242 -> [_ _ _ _ _ _ _ _ w521 _]
                tunnel: w241 -> [_ _ _ _ _ _ _ _ w516 _]
                tunnel: w239 -> [_ _ w266 w397 _ _ w458 w465 w515 _]
                tunnel: [_ _ _ _ _ _ _ _ w513 _] -> w240
                tunnel: [_ _ _ _ _ _ _ _ w511 _] -> w238
                tunnel: w237 -> [_ _ _ _ w403 _ _ w466 w510 _]
                tunnel: w236 -> [_ _ _ w402 _ _ _ _ _ w717]
                tunnel: w235 -> [_ _ _ _ _ _ _ _ w509 _]
                tunnel: [_ _ _ _ _ _ _ _ w507 _] -> w234
                tunnel: w233 -> [_ _ _ _ _ _ _ w469 w506 _]
                frame #0 {
                  # "generate initial aberration (aberr to correct)"
                  n65 = case shown="\"randomly generated\"" "?" {
                    tunnel: ["Initial Zer index" w260] -> w254
                    tunnel: ["Initial Zer coeff" w259] -> w253
                    tunnel: "max random order" -> [_ w258]
                    frame "input manually " {
                    }
                    frame "randomly generated" {
                      # "generate random zernike index and coefficient arrays"
                      n66 = call "Random Aberration Array Generator.vi"("max random order"=w258, "aberration tolerance"="aberration tolerance", "aberration threshold"="aberration threshold") -> ("Zer coeff"=w259:dbl[], "Zer index (starting from 3)"=w260:dbl[])  [unwired: 7 in]
                      "Initial Zer index (starting from 4)\nrandomly generated" <- w260
                      "Initial Zer coeff\nRandomly generated" <- w259
                    }
                  }
                }
                frame #1 {
                  # "read in offset command"
                  n67 = call-poly <vilib>:"Read From Spreadsheet File.vi"("format (%.3f)"="%.8f", "file path (dialog if empty)"="Offset command file") -> ("first row"=w263:dbl[])  [unwired: 5 in, 4 out]
                }
                frame #2 {
                  w288 = 0.0
                  # "ini zern coeff"
                  # "offset+ini command"
                  # "Zern coeff"
                  # "Zern index"
                  # "calculate the command:\nfor phase diversity"
                  n68 = Array Size(array="Zern index in 2") -> (size(s)=w286:i32)
                  n69 = call-poly <vilib>:"Ramp Pattern.vi"("start"=w288, "end"=w288, "samples"=w286) -> ("Ramp Pattern"=w285:dbl[])  [unwired: 7 in, 1 out]
                  n70 = Build Array(w285, "Zern index in 2", "Zern index in 3", "Zern index in 4", "Zern index in 5") -> (w270:T5)
                  n71 = Build Array(w285, "Zern coef in 2", "Zern coef in 3", "Zern coef in 4", "Zern coef in 5") -> (w289:T5)
                  n72 = Transpose Matrix(1:w289) -> (0:w282:T5)
                  n73 = Transpose Matrix(1:w270) -> (0:w280:T5)
                  n74 = Array Size(array=w270) -> (size(s)=w271:i32[])
                  n75 = Index Array(array=w271, index=1) -> (element=w279:i32)
                  "# of Phase" <- w279
                  n76 = stacked-sequence {
                    seq-local: [w298 _ _] -> [_ w316 w382]
                    seq-local: [w299 _ _] -> [_ w310 _]
                    seq-local: [_ w309 _] -> [_ _ w379]
                    seq-local: [w297 _ _] -> [_ w308 _]
                    tunnel: w279 -> [_ w321 _]
                    tunnel: w269 -> [w306 _ _]
                    tunnel: w268 -> [w305 w311 _]
                    tunnel: w274 -> [w304 w318 _]
                    tunnel: w283 -> [w302 _ _]
                    tunnel: w280 -> [_ w320 _]
                    tunnel: w282 -> [_ w319 _]
                    tunnel: w275 -> [w301 w317 _]
                    tunnel: [_ w315 _] -> w281
                    tunnel: w278 -> [_ w313 w380]
                    tunnel: w277 -> [_ w314 w381]
                    tunnel: w276 -> [_ w312 _]
                    tunnel: w273 -> [w300 _ _]
                    tunnel: [_ _ w378] -> w272
                    tunnel: [w298 _ _] -> w267
                    tunnel: w266 -> [_ w307 w376]
                    frame #0 {
                      n77 = call "zern2command_test.vi"("Initial haso file"=w301, "error in (no error)"=w300, "interaction matrix file"=w304, "Zern coef in"=w305, "Zern index in"=w306) -> ("error out"=w299:errorcluster, "Zern coef out"=w297:sgl[], "Offset positions"=w303:sgl[])  [unwired: 4 in]
                      n78 = Add(x=w303, y=w302) -> (x+y=w298:dbl[])
                    }
                    frame #1 {
                      n79 = for {
                        N: w321 -> [w324]
                        tunnel: w320 -> [w337] mode=indexing
                        tunnel: w319 -> [w336] mode=indexing
                        tunnel: w318 -> [w335]
                        tunnel: w317 -> [w334]
                        tunnel: w316 -> [w333]
                        tunnel: [w332] -> w315 mode=indexing
                        tunnel: w314 -> [w331]
                        tunnel: w313 -> [w330]
                        tunnel: w312 -> [w329]
                        tunnel: w311 -> [w328]
                        tunnel: w310 -> [w327]
                        tunnel: [w326] -> w309
                        tunnel: w308 -> [w323]
                        tunnel: w307 -> [w322]
                        i -> [w325]
                        n80 = stacked-sequence {
                          seq-local: [w343 _] -> [_ w362]
                          seq-local: [w339 _] -> [_ w361]
                          tunnel: w337 -> [w352 _]
                          tunnel: w336 -> [w351 _]
                          tunnel: w335 -> [w350 _]
                          tunnel: w334 -> [w349 _]
                          tunnel: w333 -> [w347 _]
                          tunnel: [w346 _] -> w332
                          tunnel: w331 -> [_ w364]
                          tunnel: w330 -> [_ w363]
                          tunnel: w329 -> [_ _]
                          tunnel: w325 -> [w345 _]
                          tunnel: w328 -> [w341 _]
                          tunnel: w327 -> [w340 _]
                          tunnel: [_ w360] -> w326
                          tunnel: w325 -> [_ _]
                          tunnel: w324 -> [_ _]
                          tunnel: w323 -> [w338 _]
                          tunnel: w322 -> [_ w357]
                          frame #0 {
                            n81 = Equal To 0?(x=w345) -> (x = 0?=w344:bool)
                            n82 = call "zern2command_test.vi"("Initial haso file"=w349, "error in (no error)"=w340, "interaction matrix file"=w350, "Zern coef in"=w351, "Zern index in"=w352) -> ("error out"=w339:errorcluster, "Zern coef out"=w342:sgl[], "Offset positions"=w348:sgl[])  [unwired: 4 in]
                            n83 = case shown="False" w344 {
                              tunnel: [w353 w354] -> w343
                              tunnel: w342 -> [w353 _]
                              tunnel: w341 -> [_ _]
                              tunnel: w338 -> [_ w354]
                              frame False {
                              }
                              frame True {
                              }
                            }
                            n84 = Add(x=w347, y=w348) -> (x+y=w346:dbl[])
                          }
                          frame #1 {
                            n85 = Number To Fractional String(number=w357, precision (6)=0) -> (F-format string=w356:string)  [unwired: 2 in]
                            n86 = Concatenate Strings(w364, w363, "_", w356, "_coeff.txt") -> (w372:string)
                            n87 = String To Path(string=w372) -> (path=w371:path)
                            n88 = Open/Create/Replace File(file path (use dialog)=w371, error in=w361, operation (0:open)=3) -> (refnum out=w368:refnum<file>, error out=w369:errorcluster)  [unwired: 3 in, 1 out]
                            n89 = Array To Spreadsheet String(array=w362, 3:"%f") -> (spreadsheet string=w359:string)  [unwired: 1 in]
                            n90 = Set File Position(refnum=w368, from (0:start)=1, error in=w369) -> (refnum out=w366:refnum<file>, error out=w365:errorcluster)  [unwired: 1 in]
                            n91 = Write to Text File(file (use dialog)=w366, text=w359, error in=w365) -> (error out=w360:errorcluster)  [unwired: 1 in, 2 out]
                          }
                        }
                      }
                    }
                    frame #2 {
                      n92 = Number To Fractional String(number=w376, precision (6)=0) -> (F-format string=w375:string)  [unwired: 2 in]
                      n93 = Concatenate Strings(w381, w380, "_", w375, "_IniAbr+offset.txt") -> (w391:string)
                      n94 = String To Path(string=w391) -> (path=w389:path)
                      n95 = Open/Create/Replace File(file path (use dialog)=w389, error in=w379, operation (0:open)=3) -> (refnum out=w386:refnum<file>, error out=w387:errorcluster)  [unwired: 3 in, 1 out]
                      n96 = Array To Spreadsheet String(array=w382, 3:"%f") -> (spreadsheet string=w393:string)  [unwired: 1 in]
                      n97 = Set File Position(refnum=w386, from (0:start)=1, error in=w387) -> (refnum out=w384:refnum<file>, error out=w383:errorcluster)  [unwired: 1 in]
                      n98 = Write to Text File(file (use dialog)=w384, text=w393, error in=w383) -> (error out=w378:errorcluster)  [unwired: 1 in, 2 out]
                    }
                  }
                }
                frame #3 {
                  # "set andor kinetics and spooling, \nstart acquire and wait for the external trigger"
                  n99 = Number To Fractional String(number=w397, precision (6)=0) -> (F-format string=w395:string)  [unwired: 2 in]
                  n100 = Concatenate Strings(w401, w400, "_PhsDiv_ToBeDeleted_", w395) -> (w398:string)
                  n101 = call "SetSpool_WaitForExtTrigger.vi"("path and name"=w398, "Kinetic Series"=w402) -> ()  [unwired: 10 in]
                }
                frame #4 {
                  # "take phase diversity pictures"
                  n102 = for {
                    N: w409 -> [_]
                    tunnel: w414 -> [w425]
                    tunnel: w413 -> [w424]
                    tunnel: w412 -> [w423]
                    tunnel: w408 -> [w422]
                    tunnel: w411 -> [w421]
                    tunnel: w410 -> [w420] mode=indexing
                    tunnel: w407 -> [w419]
                    tunnel: w406 -> [w418]
                    tunnel: [w417] -> w404
                    tunnel: [w416] -> w405
                    tunnel: w403 -> [w415]
                    n103 = stacked-sequence {
                      seq-local: [w426 _] -> [_ w435]
                      tunnel: w425 -> [_ w437]
                      tunnel: w424 -> [_ _]
                      tunnel: w423 -> [_ _]
                      tunnel: w422 -> [_ _]
                      tunnel: w421 -> [_ _]
                      tunnel: w420 -> [w427 _]
                      tunnel: w419 -> [_ w436]
                      tunnel: w418 -> [w428 _]
                      tunnel: [_ w434] -> w417
                      tunnel: [_ w433] -> w416
                      tunnel: w415 -> [w429 _]
                      frame #0 {
                        # "response time of mirror"
                        n104 = call <userlib>:"LVClass_WavefrontCorrector Move to Absolute Position.vi"("WavefrontCorrector in"=w429, "Absolute Positions"=w427, "error in (no error)"=w428) -> ("error out"=w426:errorcluster)  [unwired: 11 in, 1 out]
                        n105 = Add(x=5, y=10) -> (x+y=w430:i32)
                        n106 = Wait (ms)(milliseconds to wait=w430) -> ()  [unwired: 1 out]
                      }
                      frame #1 {
                        n107 = for {
                          N: w437 -> [_]
                          tunnel: w436 -> [w442]
                          tunnel: w435 -> [w440]
                          tunnel: [w439] -> w434
                          tunnel: [w438] -> w433
                          n108 = local read "EMCCD trigger port"() -> (w445:tag)
                          n109 = Add(x=w442, y=0.04) -> (x+y=w441:dbl)
                          n110 = Multiply(x=w441, y=1000.0) -> (x*y=w438:dbl)
                          n111 = call "trig EMCCD.vi"("error in (no error)"=w440, "exp time (ms)"=w438, "lines"=w445) -> ("error out"=w439:errorcluster)
                        }
                      }
                    }
                  }
                }
                frame #5 {
                  # "send out a trigger to EMCCD to end the aquisition."
                  n112 = local read "EMCCD trigger port"() -> (w447:tag)
                  n113 = call "trig EMCCD.vi"("exp time (ms)"=w446, "lines"=w447) -> ()  [unwired: 1 in, 1 out]
                }
                frame #6 {
                  w454 = 0
                  # "save phase diversity pictures:\npictures per phase*number of phases (Eg: 2*5=10 pictures in this file)"
                  n114 = Number To Fractional String(number=w458, precision (6)=w454) -> (F-format string=w453:string)  [unwired: 2 in]
                  n115 = Concatenate Strings(w459, "_", w453) -> (w449:string)
                  "phase diversity file name" <- w449
                  n116 = Concatenate Strings(w449, ".tif") -> (w450:string)
                  n117 = Concatenate Strings(w457, w450) -> (w452:string)
                  n118 = call <userlib>:"SaveAsTiff.vi"("path"=w452, "palette"="C:\\Program Files\\Andor SOLIS\\GREY.PAL", "position"=w454, "type"=1) -> ()  [unwired: 10 in, 2 out]
                }
                frame #7 {
                  # "offset+ini path and name no.tif"
                  # "groundtruth path and name no.tif"
                  n119 = stacked-sequence {
                    seq-local: [w471 _ _ _] -> [_ w484 _ _]
                    seq-local: [_ _ w487 _] -> [_ _ _ w500]
                    tunnel: w468 -> [w476 _ w493 _]
                    tunnel: w467 -> [w475 _ w492 _]
                    tunnel: w465 -> [w474 _ w491 _]
                    tunnel: w463 -> [w473 _ w490 _]
                    tunnel: w462 -> [_ _ w489 _]
                    tunnel: w466 -> [w472 _ w488 _]
                    tunnel: w469 -> [_ w485 _ w503]
                    tunnel: [_ w481 _ _] -> w460
                    tunnel: w464 -> [w470 _ _ _]
                    tunnel: [_ _ _ w498] -> w461
                    frame #0 {
                      # "take a picture of groundtruth"
                      n120 = Number To Fractional String(number=w474, precision (6)=0) -> (F-format string=w477:string)  [unwired: 2 in]
                      n121 = Concatenate Strings(w476, w475, "_grdtrth_", w477) -> (w471:string)
                      n122 = call "Apply DM command and take picture.vi"("WavefrontCorrector in"=w472, "Offset positions"=w470, "trigger time (ms)"=w473, "# of pictures"=1, "path and file name, no .tif at the end"=w471) -> ()  [unwired: 6 in, 1 out]
                    }
                    frame #1 {
                      # "calculate imq of groundtruth"
                      n123 = Concatenate Strings(w484, ".tif") -> (w482:string)
                      n124 = call "MATLAB image quality metrics.vi"("Background Value"=w485, "File Path and Name w/.tif"=w482, "Metrics Type"="Metrics Type") -> ("image quality"=w481:dbl)  [unwired: 8 in]
                    }
                    frame #2 {
                      # "take a picture of offset+ini abbr"
                      n125 = Number To Fractional String(number=w491, precision (6)=0) -> (F-format string=w494:string)  [unwired: 2 in]
                      n126 = Concatenate Strings(w493, w492, "_abbr_", w494) -> (w487:string)
                      n127 = call "Apply DM command and take picture.vi"("WavefrontCorrector in"=w488, "Offset positions"=w489, "trigger time (ms)"=w490, "# of pictures"=1, "path and file name, no .tif at the end"=w487) -> ()  [unwired: 6 in, 1 out]
                    }
                    frame #3 {
                      # "calculate imq of offset+ini"
                      n128 = local read "Metrics Type"() -> (w499:T3)
                      n129 = Concatenate Strings(w500, ".tif") -> (w501:string)
                      n130 = call "MATLAB image quality metrics.vi"("Background Value"=w503, "File Path and Name w/.tif"=w501, "Metrics Type"=w499) -> ("image quality"=w498:dbl)  [unwired: 8 in]
                    }
                  }
                }
                frame #8 {
                  # "run matlab correction?"
                  n131 = case shown="True" w516 {
                    tunnel: w522 -> [_ w544]
                    tunnel: w523 -> [_ w543]
                    tunnel: w521 -> [_ w542]
                    tunnel: w520 -> [w524 w541]
                    tunnel: w518 -> [_ w528]
                    tunnel: w519 -> [_ w540]
                    tunnel: w517 -> [_ w539]
                    tunnel: w515 -> [_ w538]
                    tunnel: w514 -> [_ _]
                    tunnel: [0 w537] -> w513
                    tunnel: w512 -> [_ w536]
                    tunnel: [errorcluster {"status"=FALSE, "code"=0, "source"=""} ("Error out 2") w535] -> w511
                    tunnel: w510 -> [_ w534]
                    tunnel: w509 -> [_ w533]
                    tunnel: w508 -> [_ _]
                    tunnel: [w524 w532] -> w507
                    tunnel: w506 -> [_ w531]
                    tunnel: w505 -> [_ w529]
                    tunnel: w504 -> [_ w527]
                    frame False {
                    }
                    frame True {
                      # "matlab recons Zern"
                      # "matlab reconstructed Zern"
                      n132 = stacked-sequence {
                        seq-local: [_ _ _ _ w659 _ _ _ _ _ _] -> [_ _ _ _ _ w666 _ _ _ _ _]
                        seq-local: [_ _ w647 _ _ _ _ _ _ _ _] -> [_ _ _ w654 _ _ _ _ _ _ _]
                        seq-local: [_ _ _ w656 _ _ _ _ _ _ _] -> [_ _ _ _ w660 _ _ _ _ _ _]
                        seq-local: [_ w639 _ _ _ _ _ _ _ _ _] -> [_ _ _ _ _ _ _ _ _ _ w706]
                        seq-local: [_ _ _ _ _ _ w671 _ _ _ _] -> [_ _ _ _ _ _ _ w684 _ _ _]
                        seq-local: [w551 _ _ _ _ _ _ _ _ _ _] -> [_ _ _ _ _ _ _ _ _ _ _]
                        seq-local: [w550 _ _ _ _ _ _ _ _ _ _] -> [_ _ _ _ _ _ w669 _ _ _ _]
                        tunnel: w544 -> [w552 w642 _ _ _ _ _ _ _ w695 _]
                        tunnel: w543 -> [w549 w641 _ _ _ _ _ _ _ w694 _]
                        tunnel: w542 -> [w548 _ _ _ _ _ w679 _ _ _ _]
                        tunnel: w541 -> [w547 _ _ _ w661 _ w678 _ _ _ _]
                        tunnel: w528 -> [_ _ _ w658 _ w668 _ w686 w692 _ _]
                        tunnel: w539 -> [_ _ w648 _ _ _ _ _ _ _ _]
                        tunnel: [_ _ _ w657 _ _ _ _ _ _ _] -> _
                        tunnel: w540 -> [_ _ _ w657 _ _ _ w685 _ _ _]
                        tunnel: w538 -> [w554 w640 _ _ _ _ _ _ _ w696 _]
                        tunnel: [w553 _ _ _ _ _ _ _ _ _ _] -> w537
                        tunnel: w536 -> [_ _ w649 _ _ _ _ _ _ _ _]
                        tunnel: [_ _ _ _ _ _ _ w683 _ _ _] -> w535
                        tunnel: w534 -> [_ _ w650 _ w662 _ w673 _ _ _ _]
                        tunnel: w533 -> [_ w643 _ _ _ _ _ _ _ _ w704]
                        tunnel: [_ _ _ _ _ _ w670 _ _ _ _] -> w532
                        tunnel: w531 -> [w556 _ _ _ _ _ _ _ _ _ _]
                        tunnel: 2 -> [w557 _ _ _ _ _ _ _ _ _ _]
                        tunnel: w529 -> [w555 _ _ _ _ _ _ _ _ _ _]
                        tunnel: w528 -> [w546 _ _ _ _ _ _ _ _ _ _]
                        tunnel: w527 -> [w545 _ _ _ _ _ _ _ _ _ _]
                        frame #0 {
                          n133 = while {
                            shift-right: [w573] -> _
                            shift-left: w557 -> [w574]
                            tunnel: w556 -> [w571]
                            tunnel: w555 -> [w570]
                            tunnel: w554 -> [w567]
                            tunnel: [w566] -> w553
                            tunnel: w552 -> [w565]
                            tunnel: [w564] -> w551
                            tunnel: [w563] -> w550
                            tunnel: w549 -> [w562]
                            tunnel: w548 -> [w561]
                            tunnel: w547 -> [w560]
                            tunnel: w546 -> [w559]
                            tunnel: w545 -> [w558]
                            stop <- w568 stop-if-true
                            n134 = stacked-sequence {
                              seq-local: [_ w606 _ _] -> [_ _ w627 _]
                              seq-local: [w577 _ _ _] -> [_ w614 _ _]
                              seq-local: [w576 _ _ _] -> [_ w613 _ _]
                              tunnel: w574 -> [w582 w607 _ w637]
                              tunnel: [_ _ _ w636] -> w573
                              tunnel: [_ _ _ w635] -> w572
                              tunnel: w571 -> [w581 _ w630 _]
                              tunnel: w570 -> [_ _ w629 _]
                              tunnel: [_ _ w628 _] -> w569
                              tunnel: w567 -> [w580 w608 _ _]
                              tunnel: [w579 _ _ _] -> w566
                              tunnel: w565 -> [w578 w610 _ _]
                              tunnel: [w577 _ _ _] -> w564
                              tunnel: [w576 _ _ _] -> w563
                              tunnel: w562 -> [w575 w609 _ _]
                              tunnel: w561 -> [_ w615 _ _]
                              tunnel: w560 -> [_ w612 _ _]
                              tunnel: w559 -> [_ w611 _ _]
                              tunnel: w558 -> [_ w605 _ _]
                              frame #0 {
                                # "MATLAB does the reconstruction, written by Min Guo"
                                # "other parameters are default in this VI"
                                n135 = Number To Fractional String(number=w580, precision (6)=0) -> (F-format string=w592:string)  [unwired: 2 in]
                                n136 = Concatenate Strings(w575, "_", w592) -> (w583:string)
                                n137 = String To Path(string=w578) -> (path=w599:path)
                                n138 = Concatenate Strings(w578, w583) -> (w598:string)
                                n139 = String To Path(string=w598) -> (path=w597:path)
                                n140 = call "recon_zern_fileIO_MATLAB.vi"("Number of Phase"=w582, "Number for average"="Number for average 2", "Crop Size of image"="Crop Size of image 2", "Background Value"=w581, "Zernike Order"="Zernike Order 2", "Use GPU"="Use GPU 2", "Iteration Number"="Iteration Number 2", "File Name"=w583, "Gamma Value"="Gamma Value 2", "Path In"=w599, "Show Input"="Show Input 2", "Path Out"=w597, "Show Recon"="Show Recon 2") -> ("Zern coef out"=w595:sgl[], "RMSE Value"=w579:dbl, "error out"=w577:errorcluster)  [unwired: 3 in, 1 out]
                                n141 = case shown="True" "Keep Reconstructed Defocus component? 2" {
                                tunnel: w595 -> [w600 w604]
                                tunnel: [w600 w601] -> w576
                                frame False {
                                }
                                frame True {
                                n142 = Replace Array Subset(array=w604, new element=0.0, index=2) -> (w601:sgl[])
                                }
                                }
                              }
                              frame #1 {
                                w617 = 0
                                w626 = 1
                                # "get correction command\ntake a picture"
                                n143 = call-poly <vilib>:"Ramp Pattern.vi"("start"=w626, "end"=32, "delta"=w626) -> ("Ramp Pattern"=w624:dbl[])  [unwired: 6 in, 2 out]
                                n144 = call "zern2command_test.vi"("Initial haso file"=w605, "error in (no error)"=w614, "interaction matrix file"=w615, "Zern coef in"=w613, "Zern index in"=w624) -> ("Offset positions"=w623:sgl[])  [unwired: 4 in, 2 out]
                                n145 = Add(x=w612, y=w623) -> (x+y=w622:dbl[])
                                n146 = Number To Fractional String(number=w608, precision (6)=w617) -> (F-format string=w619:string)  [unwired: 2 in]
                                n147 = Number To Fractional String(number=w607, precision (6)=w617) -> (F-format string=w616:string)  [unwired: 2 in]
                                n148 = Concatenate Strings(w610, w609, "_", w616, "ImgCorr_", w619) -> (w606:string)
                                n149 = call "Apply DM command and take picture.vi"("Offset positions"=w622, "trigger time (ms)"=w611, "# of pictures"=1, "path and file name, no .tif at the end"=w606) -> ()  [unwired: 7 in, 1 out]
                              }
                              frame #2 {
                                n150 = local read "Metrics Type"() -> (w632:T3)
                                n151 = Concatenate Strings(w627, ".tif") -> (w633:string)
                                n152 = call "MATLAB image quality metrics.vi"("Background Value"=w630, "File Path and Name w/.tif"=w633, "Metrics Type"=w632) -> ("image quality"=w631:dbl)  [unwired: 8 in]
                                n153 = Greater?(x=w631, y=w629) -> (0:w628:bool)
                              }
                              frame #3 {
                                n154 = Increment(x=w637) -> (x+1=w636:i32)
                                n155 = Greater?(x=w636, y=5) -> (0:w635:bool)
                              }
                            }
                            n156 = Or(x=w569, y=w572) -> (x .or. y?=w568:bool)
                          }
                        }
                        frame #1 {
                          # "set andor kinetics and spooling, \nstart acquire and wait for the external trigger"
                          n157 = Number To Fractional String(number=w640, precision (6)=0) -> (F-format string=w644:string)  [unwired: 2 in]
                          n158 = Concatenate Strings(w642, w641, "_Corr_ToBeDeleted_", w644) -> (w639:string)
                          n159 = call "SetSpool_WaitForExtTrigger.vi"("path and name"=w639, "Kinetic Series"=w643) -> ()  [unwired: 10 in]
                        }
                        frame #2 {
                          # "groundtruth command"
                          # "response time of mirror"
                          n160 = call <userlib>:"LVClass_WavefrontCorrector Move to Absolute Position.vi"("WavefrontCorrector in"=w650, "Absolute Positions"=w649, "error in (no error)"=w648) -> ("error out"=w647:errorcluster)  [unwired: 11 in, 1 out]
                          n161 = Add(x=5, y=10) -> (x+y=w651:i32)
                          n162 = Wait (ms)(milliseconds to wait=w651) -> ()  [unwired: 1 out]
                        }
                        frame #3 {
                          # "take offset/groundtruth picture, only one"
                          n163 = local read "EMCCD trigger port"() -> (w655:tag)
                          n164 = call "trig EMCCD.vi"("error in (no error)"=w654, "exp time (ms)"=w658, "lines"=w655) -> ("error out"=w656:errorcluster)
                        }
                        frame #4 {
                          # "aberrated picture command"
                          # "response time of mirror"
                          n165 = call <userlib>:"LVClass_WavefrontCorrector Move to Absolute Position.vi"("WavefrontCorrector in"=w662, "Absolute Positions"=w661, "error in (no error)"=w660) -> ("error out"=w659:errorcluster)  [unwired: 11 in, 1 out]
                          n166 = Add(x=5, y=10) -> (x+y=w663:i32)
                          n167 = Wait (ms)(milliseconds to wait=w663) -> ()  [unwired: 1 out]
                        }
                        frame #5 {
                          # "take offset+initial aberr picture, only one"
                          n168 = local read "EMCCD trigger port"() -> (w667:tag)
                          n169 = call "trig EMCCD.vi"("error in (no error)"=w666, "exp time (ms)"=w668, "lines"=w667) -> ()  [unwired: 1 out]
                        }
                        frame #6 {
                          w682 = 1
                          # "correction command"
                          # "response time of mirror"
                          n170 = call-poly <vilib>:"Ramp Pattern.vi"("start"=w682, "end"=32, "delta"=w682) -> ("Ramp Pattern"=w680:dbl[])  [unwired: 6 in, 2 out]
                          n171 = call "zern2command_test.vi"("interaction matrix file"=w679, "Zern coef in"=w669, "Zern index in"=w680) -> ("error out"=w672:errorcluster, "Offset positions"=w677:sgl[])  [unwired: 6 in, 1 out]
                          n172 = Add(x=w678, y=w677) -> (x+y=w670:dbl[])
                          n173 = call <userlib>:"LVClass_WavefrontCorrector Move to Absolute Position.vi"("WavefrontCorrector in"=w673, "Absolute Positions"=w670, "error in (no error)"=w672) -> ("error out"=w671:errorcluster)  [unwired: 11 in, 1 out]
                          n174 = Add(x=5, y=10) -> (x+y=w674:i32)
                          n175 = Wait (ms)(milliseconds to wait=w674) -> ()  [unwired: 1 out]
                        }
                        frame #7 {
                          # "corrected pictures"
                          n176 = for {
                            N: w685 -> [_]
                            tunnel: w686 -> [w689]
                            shift-right: [w687] -> w683
                            shift-left: w684 -> [w688]
                            n177 = local read "EMCCD trigger port"() -> (w690:tag)
                            n178 = call "trig EMCCD.vi"("error in (no error)"=w688, "exp time (ms)"=w689, "lines"=w690) -> ("error out"=w687:errorcluster)
                          }
                        }
                        frame #8 {
                          # "one more trigger to end picture acquisition"
                          n179 = local read "EMCCD trigger port"() -> (w691:tag)
                          n180 = call "trig EMCCD.vi"("exp time (ms)"=w692, "lines"=w691) -> ()  [unwired: 1 in, 1 out]
                        }
                        frame #9 {
                          w699 = 0
                          # "save:\none groundtruth picture\none offset+abrr picture\nPictures per phase*corrected picture"
                          n181 = Number To Fractional String(number=w696, precision (6)=w699) -> (F-format string=w698:string)  [unwired: 2 in]
                          n182 = Concatenate Strings(w694, "_grdtrth_abrr_Corr_", w698, ".tif") -> (w703:string)
                          "Corrected Picture name" <- w703
                          n183 = Concatenate Strings(w695, w703) -> (w697:string)
                          n184 = call <userlib>:"SaveAsTiff.vi"("path"=w697, "palette"="C:\\Program Files\\Andor SOLIS\\GREY.PAL", "position"=w699, "type"=1) -> ()  [unwired: 10 in, 2 out]
                        }
                        frame #10 {
                          n185 = case shown="True" TRUE {
                            tunnel: w706 -> [_ w708]
                            tunnel: w704 -> [_ w707]
                            frame False {
                            }
                            frame True {
                              # "delete spooling data"
                              n186 = for {
                                N: w707 -> [_]
                                tunnel: w708 -> [w715]
                                i -> [w713]
                                n187 = Number To Fractional String(number=w713, precision (6)=0) -> (F-format string=w711:string)  [unwired: 2 in]
                                n188 = Concatenate Strings(w715, "000000000", w711, ".dat") -> (w710:string)
                                n189 = String To Path(string=w710) -> (path=w716:path)
                                n190 = Delete(path (use dialog)=w716) -> ()  [unwired: 4 in, 3 out]
                              }
                            }
                          }
                        }
                      }
                    }
                  }
                }
                frame #9 {
                  # "delete spooling data of phase diversity"
                  n191 = case shown="True" TRUE {
                    tunnel: w719 -> [_ w721]
                    tunnel: w717 -> [_ w720]
                    frame False {
                    }
                    frame True {
                      n192 = for {
                        N: w720 -> [_]
                        tunnel: w721 -> [w724]
                        i -> [w723]
                        n193 = Number To Fractional String(number=w723, precision (6)=0) -> (F-format string=w726:string)  [unwired: 2 in]
                        n194 = Concatenate Strings(w724, "000000000", w726, ".dat") -> (w722:string)
                        n195 = String To Path(string=w722) -> (path=w729:path)
                        n196 = Delete(path (use dialog)=w729) -> ()  [unwired: 4 in, 3 out]
                      }
                    }
                  }
                }
              }
            }
          }
          frame #3 {
            # "shut down shutter of 488nm laser"
            n197 = invoke class="MG17Motor" method="SC_Disable"(reference=w733, "lChanID"=w732) -> (reference out=w731:refnum<k7>, "lChanID"=w730:i32)  [unwired: 2 in, 2 out]
          }
          frame #4 {
            # "save the RMS of (calculated zer-real zer)"
            n198 = Concatenate Strings(w736, w735, "_RMSE.txt") -> (w741:string)
            n199 = String To Path(string=w741) -> (path=w740:path)
            n200 = Number To Fractional String(number=w737) -> (F-format string=w738:string[])  [unwired: 3 in]
            n201 = Write to Text File(file (use dialog)=w740, text=w738) -> (error out=w734:errorcluster)  [unwired: 2 in, 2 out]
          }
        }
        n202 = Merge Errors(w182, w181, w176) -> (w175:errorcluster)
        "Error out" <- w175
        n203 = Unbundle(w175) -> ("status"=w171:bool)  [unwired: 2 out]
        n204 = case shown="True" w171 {
          tunnel: [w197 w198] -> w174
          tunnel: w171 -> [w196 w198]
          frame False {
            n205 = Not(x=w196) -> (.not. x?=w197:bool)
          }
          frame True {
          }
        }
        n206 = Or(x=w174, y="?") -> (x .or. y?=w172:bool)
      }
    }
    frame #4 {
      # "# of z slices"
      # "open 488 shutter\napply correction matrix to DM\nset spooling\ntake picture from Z_top to Z_bottom in a step of delta_Z, show current Z\nall these pictures in one .tif file\nturn off shutter"
      n207 = Multiply(x="Z scanning range (um)", y=2.0) -> (x*y=w749:dbl)
      n208 = Divide(x=w749, y="Z scanning step (um)") -> (x/y=w748:dbl)
      n209 = Increment(x=w748) -> (x+1=w747:dbl)
      n210 = stacked-sequence {
        seq-local: [w756 _ _ _ _ _ _ _] -> [_ _ _ _ _ _ _ _]
        seq-local: [w755 _ _ _ _ _ _ _] -> [_ _ _ _ _ _ _ _]
        tunnel: w754 -> [w758 _ _ _ _ _ _ w825]
        tunnel: w753 -> [w757 _ _ _ _ _ _ w824]
        tunnel: w752 -> [_ w760 _ _ _ _ _ _]
        tunnel: w751 -> [_ w759 _ _ _ _ _ _]
        tunnel: w747 -> [_ _ w763 w769 _ _ w806 _]
        tunnel: w746 -> [_ _ w762 _ _ w800 w805 _]
        tunnel: w745 -> [_ _ w761 _ _ w799 w804 _]
        tunnel: "Z scanning range (um)" -> [_ _ _ w767 _ _ _ _]
        tunnel: "Z scanning step (um)" -> [_ _ _ w768 _ _ _ _]
        tunnel: w742 -> [_ _ _ w766 w795 _ _ _]
        frame #0 {
          n211 = invoke class="MG17Motor" method="SC_Enable"(reference=w758, "lChanID"=w757) -> (reference out=w756:refnum<k7>, "lChanID"=w755:i32)  [unwired: 2 in, 2 out]
        }
        frame #1 {
          n212 = call <userlib>:"LVClass_WavefrontCorrector Move to Absolute Position.vi"("WavefrontCorrector in"=w759, "Absolute Positions"=w760) -> ()  [unwired: 12 in, 2 out]
        }
        frame #2 {
          n213 = Concatenate Strings(w762, w761, "_3D") -> (w764:string)
          n214 = call "SetSpool_WaitForExtTrigger.vi"("path and name"=w764, "Kinetic Series"=w763) -> ()  [unwired: 10 in]
        }
        frame #3 {
          n215 = for {
            N: w769 -> [_]
            tunnel: w768 -> [w773]
            tunnel: w767 -> [w772]
            tunnel: w766 -> [w771]
            i -> [w770]
            n216 = stacked-sequence {
              tunnel: w773 -> [w778 _ _ _]
              tunnel: w772 -> [w781 _ _ _]
              tunnel: w771 -> [_ _ _ w793]
              tunnel: w770 -> [w779 _ _ _]
              frame #0 {
                # "10 step=1um"
                # "move to z"
                n217 = local read "Z for correction (um) (10 steps=1um)"() -> (w782:dbl)
                n218 = local read "ASI stage VISA resource name"() -> (w783:refnum<visa-resource-name>)
                n219 = Subtract(x=w782, y=w781) -> (x-y=w780:dbl)
                n220 = Multiply(x=w778, y=w779) -> (x*y=w777:dbl)
                n221 = Add(x=w780, y=w777) -> (x+y=w776:dbl)
                n222 = Multiply(x=w776, y=10) -> (x*y=w774:dbl)
                n223 = Number To Decimal String(number=w774) -> (decimal integer string=w785:string)  [unwired: 1 in]
                n224 = Concatenate Strings("move z=", w785) -> (w784:string)
                n225 = call "WriteCmd.vi"("Command"=w784, "VISA resource name"=w783) -> ()  [unwired: 1 in, 1 out]
              }
              frame #1 {
                n226 = Wait (ms)(milliseconds to wait=300) -> ()  [unwired: 1 out]
              }
              frame #2 {
                # "show z coordinate"
                n227 = local read "ASI stage VISA resource name"() -> (w791:refnum<visa-resource-name>)
                n228 = call "WriteCmd.vi"("Command"="where z", "VISA resource name"=w791) -> ("error"=w792:errorcluster)  [unwired: 1 in]
                n229 = VISA Read(VISA resource name=w791, byte count=100, error in (no error)=w792) -> (read buffer=→"Current Z in step":string)  [unwired: 3 out]
              }
              frame #3 {
                # "send a trigger to take picture"
                n230 = local read "EMCCD trigger port"() -> (w794:tag)
                n231 = call "trig EMCCD.vi"("exp time (ms)"=w793, "lines"=w794) -> ()  [unwired: 1 in, 1 out]
              }
            }
          }
        }
        frame #4 {
          # "send a trigger to end the acquisition"
          n232 = local read "EMCCD trigger port"() -> (w796:tag)
          n233 = call "trig EMCCD.vi"("exp time (ms)"=w795, "lines"=w796) -> ()  [unwired: 1 in, 1 out]
        }
        frame #5 {
          # "save .tif"
          n234 = Concatenate Strings(w800, w799, "_3D.tif") -> (w797:string)
          n235 = call <userlib>:"SaveAsTiff.vi"("path"=w797, "palette"="C:\\Program Files\\Andor SOLIS\\GREY.PAL", "position"=0, "type"=1) -> ()  [unwired: 10 in, 2 out]
        }
        frame #6 {
          # "delete spooling data"
          n236 = for {
            N: w806 -> [_]
            tunnel: w805 -> [w815]
            tunnel: w804 -> [w814]
            i -> [w807]
            n237 = Number To Decimal String(number=w807) -> (decimal integer string=w813:string)  [unwired: 1 in]
            n238 = String Length(string=w813) -> (length=w811:i32)
            n239 = Subtract(x=10, y=w811) -> (x-y=w810:i32)
            n240 = for {
              N: w810 -> [_]
              shift-right: [w823] -> w808
              shift-left: "_3D" -> [w822]
              n241 = Concatenate Strings(w822, "0") -> (w823:string)
            }
            n242 = Number To Fractional String(number=w807, precision (6)=0) -> (F-format string=w818:string)  [unwired: 2 in]
            n243 = Concatenate Strings(w815, w814, w808, w818, ".dat") -> (w816:string)
            n244 = String To Path(string=w816) -> (path=w820:path)
            n245 = Delete(path (use dialog)=w820) -> ()  [unwired: 4 in, 3 out]
          }
        }
        frame #7 {
          # "488 shutter off"
          n246 = invoke class="MG17Motor" method="SC_Disable"(reference=w825, "lChanID"=w824) -> ()  [unwired: 2 in, 4 out]
        }
      }
    }
    frame #5 {
      n247 = case shown="True" "Turn off EMCCD when finished?" {
        frame False {
        }
        frame True {
          n248 = flat-sequence {
            frame #0 {
              n249 = call <userlib>:"CoolerOFF.vi"() -> ()  [unwired: 2 in, 2 out]
            }
            frame #1 {
              # "shut down EMCCD"
              n250 = call <userlib>:"ShutDown.vi"() -> ()  [unwired: 2 in, 2 out]
            }
          }
        }
      }
    }
    frame #6 {
      # "shut down casao"
      n251 = call <userlib>:"LVClass_WavefrontCorrector dtor.vi"("WavefrontCorrector in"=w830, "error in (no error)"=w828) -> ("error out"=w827:errorcluster)  [unwired: 12 in, 1 out]
      n252 = call <userlib>:"LVClass_WavefrontCorrectorSet dtor.vi"("WavefrontCorrectorSet in"=w829, "error in (no error)"=w827) -> ()  [unwired: 12 in, 2 out]
      n253 = invoke class="MG17Motor" method="StopCtrl"(reference=w831) -> ()  [unwired: 2 in, 3 out]
    }
  }
